vi "StandAlone_TransientDataCollection.vi"() -> ()   [LabVIEW 2019]
uses:
  <instrlib>/niScope/Controls/niScope vertical coupling.ctl
  <vilib>/Utility/file.llb/Write Delimited Spreadsheet (string).vi
  <instrlib>/niScope/Configure/Trigger/niScope Configure Trigger Software.vi
  <instrlib>/niScope/Acquire/Fetch/niScope Multi Fetch Binary 16.vi
panel:
  in  "ON/OFF":bool
  in  "Using an RF Source?":bool
  in  "power (dBm)":dbl
  in  "frequency (GHz)":dbl
  in  "Apply RF Source Changes":bool
  in  "RF Source":refnum<visa-resource-name>
  out "current limit ind":dbl
  out "Channel 0 Reference Values":dbl[](array[numeric])
  out "CHANNEL 7 NAME":string
  out "CHANNEL 6 NAME":string
  out "CHANNEL 5 NAME":string
  out "CHANNEL 4 NAME":string
  out "CHANNEL 3 NAME":string
  out "CHANNEL 2 NAME":string
  out "CHANNEL 1 NAME":string
  out "CHANNEL 0 NAME":string
  out "RUN_FOLDER":path
  out "RESTART PROGRAM SOON (DATACOLLECT)":bool
  out "Sample Rate IND":dbl
  out "Channel To Mitigate (0-7) IND":i32
  out "Collecting Data":bool
  out "RESTART PROGRAM SOON (DATASTORE)":bool
  out "Threshold Value":dbl
  out "Num Loop 4 Reset Graph":i32
  out "Channel Graph Cumulative 7":dbl[](graph)
  out "Channel Graph Cumulative 6":dbl[](graph)
  out "Channel Graph Cumulative 5":dbl[](graph)
  out "Channel Graph Cumulative 4":dbl[](graph)
  out "Channel Graph Cumulative 3":dbl[](graph)
  out "Channel Graph Cumulative 2":dbl[](graph)
  out "Channel Graph Cumulative 1":dbl[](graph)
  out "Channel Graph Cumulative 0":dbl[](graph)
  out "Channel Graph 7":dbl[](graph)
  out "Channel Graph 6":dbl[](graph)
  out "Channel Graph 5":dbl[](graph)
  out "Channel Graph 4":dbl[](graph)
  out "Channel Graph 3":dbl[](graph)
  out "Channel Graph 2":dbl[](graph)
  out "Channel Graph 1":dbl[](graph)
  out "Channel Graph 0":dbl[](graph)
  in  "Channel To Mitigate (0-7)":i32
  out "Last Point Fetched":i32
  out "Total Points Fetched":i32
  out "NUMBER SAMPLES":i32
  out "XINC":dbl
  out "Nominal Current IND":dbl
  out "Percent Threshold IND":dbl
  out "EXCEED THRESHOLD":bool
  out "EXCEED DURATION":bool
  out "Over Threshold Number":i32
  out "number of resets":i32
  out "ENABLE STATE":bool
  in  "DC Power On":bool
  in  "TRANSIENT TIME DURATION (ms)":dbl=500.0
  in  "milliseconds to wait":u32
  in  "vertical coupling":T1=1 items=["AC", "DC", "Ground"]
  in  "min record length":i32=100000
  in  "INTIALIZE SCOPE":bool
  in  "50 ohm vertical range (V)":dbl=10.0 caption="50 ohm vertical range" format="%.2f"
  in  "Channel 0 50 ohms?":bool
  out "wfm info IND":T2(array[cluster]) caption="wfm info" {"reserved2" format="%.2f"; "reserved1" format="%.2f"; "offset" format="%^.3e"; "gain" format="%^.3e"; "xIncrement" format="%^.3e"; "relativeInitialX" format="%^.3e"; "absoluteInitialX" format="%^.3e"}
  out "AUTOMITIGATION ENABLED IND":bool
  in  "AUTOMITIGATION ENABLED":bool
  out "Vertical Range (V) IND":dbl=30.0 caption="Vertical Range (V)" format="%_3g"
  out "channels IND":string="0" caption="channels"
  out "Min. Sample Rate IND":dbl=50000.0 caption="Min. Sample Rate" format="%#_6p"
  in  "Ion (ex. Kr)":string
  in  "Effective LET":string
  in  "Board Number":string
  in  "DUT":string
  in  "Beam On?":bool
  in  "Percent Threshold":dbl
  in  "Nominal Mitigation Value":dbl
  out "Number Of Channels":i32
  in  "Plot Data?":bool=TRUE
  out "CURRENTPATH":path
  out "FOLDERCREATED":bool=TRUE
  out "IndicatorOutputs":cluster{"Run Information":string, string}
  out "Latchup_or_Transient":bool
  out "BinaryRefObjects":T3
  out "OscopeParamPath":path
  out "INITIALIZED":bool
  in  "APPLYPATH":bool
  in  "INPUTPATH":path=path "C:/Campaigns/LBNL_May_2025"
  in  "Max Points per Fetch":i32=-1
  in  "channels":string="Current,Vin,Vout1,Vout2,PowerGood1_2,EN1,EN2,BeamSignal" caption="channels (comma separated)"
  in  "Oscilloscope":refnum<k15>="PXIe-5172"
  in  "Min. Sample Rate":dbl=50000.0 format="%#_6p"
  in  "Vertical Range (V)":dbl=30.0 format="%_3g"
  out "RECORDING DATA":bool
  in  "BEGIN RECORDING":bool
  out "Present Mitigation Information":string
  out "NIDCPOWER_VOLT_CONF":dbl caption="voltage level IND" format="%.6p"
  out "NIDCPOWER_CHAN_CONF":string
  in  "NIDCPOWER_VOLT":dbl caption="voltage level" format="%.6p"
  in  "NIDCPOWER_CHAN":string="0"
  in  "resource name":refnum<k15>="Slot_4_PXIe4139" caption="DC Power PSU"
  in  "CHANGE MITIGATION":bool
  in  "Mitigation":u16(ring) items=["None", "Hardware", "PowerCycle", "EnableCircuit"]
  out "FINISH PROGRAM":bool
  in  "FORCED RESET":bool
  out "POWER STATE":bool
  in  "Channels to Parallelize (if selected)":u16(ring) items=["I1+I2", "ALL", "I2+I3"]
  out "Present Channel Configuration":string
  out "Channels Configured and Values":string[][](array[string])
  in  "Combination":u16(ring) items=["OFF", "SERIES", "PARALLEL"]
  in  "PSU":refnum<visa-resource-name>="USB0::0x05E6::0x2230::802901012767010005::INSTR"
  in  "Current Limit Channel 3":dbl
  in  "Current Limit Channel 2":dbl
  in  "Current Limit Channel 1":dbl
  in  "Voltage Channel 3":dbl
  in  "Voltage Channel 2":dbl
  in  "Voltage Channel 1":dbl
  in  "stop":bool
  in  "APPLY POWER SETTINGS":bool
  in  "POWER ON":bool
  # "11 In order, name all of the channels 0-7"
  # "3 press the white arrow"
  # "10 this is the maximum. Make it smaller for better resolution"
  # "OSCILLOSCOPE BLOCK"
  # "DATA BLOCK"
  # "5 enter where the data"
  # "Use this for step three"
  # "9 if needed"
  # "12 set the scope to the configurations from steps 9-11 on device"
  # "Nothing behind here"
  # "6 enter in values before each run"
  # "need to fix this"
  # "13,16 begin recording data"
  # "1"
  # "17 end program"
  # "2"
  # "14,15 saying the beam is on or could just have the TTL logic"
  # "7 enter in values before each run"
  # "POWER BLOCK"
  # "NI DCPower"
  # "NOTE THAT VISA POWER HAS THE NI DC POWER TURN OFF AS WELL"
  # "4"
  # "Current"
  # "8 power on device"
  # "Ignore all of this"
  # "7 power on device"
  # "7 power on device"
  # "7 power on device"
  # "7 power on device"
  # "7 power on device"
  # "7 power on device"
  # "7 power on device"
  # "7 power on device"
  # "7 power on device"
  # "7 power on device"
  # "7 power on device"
  # "7 power on device"
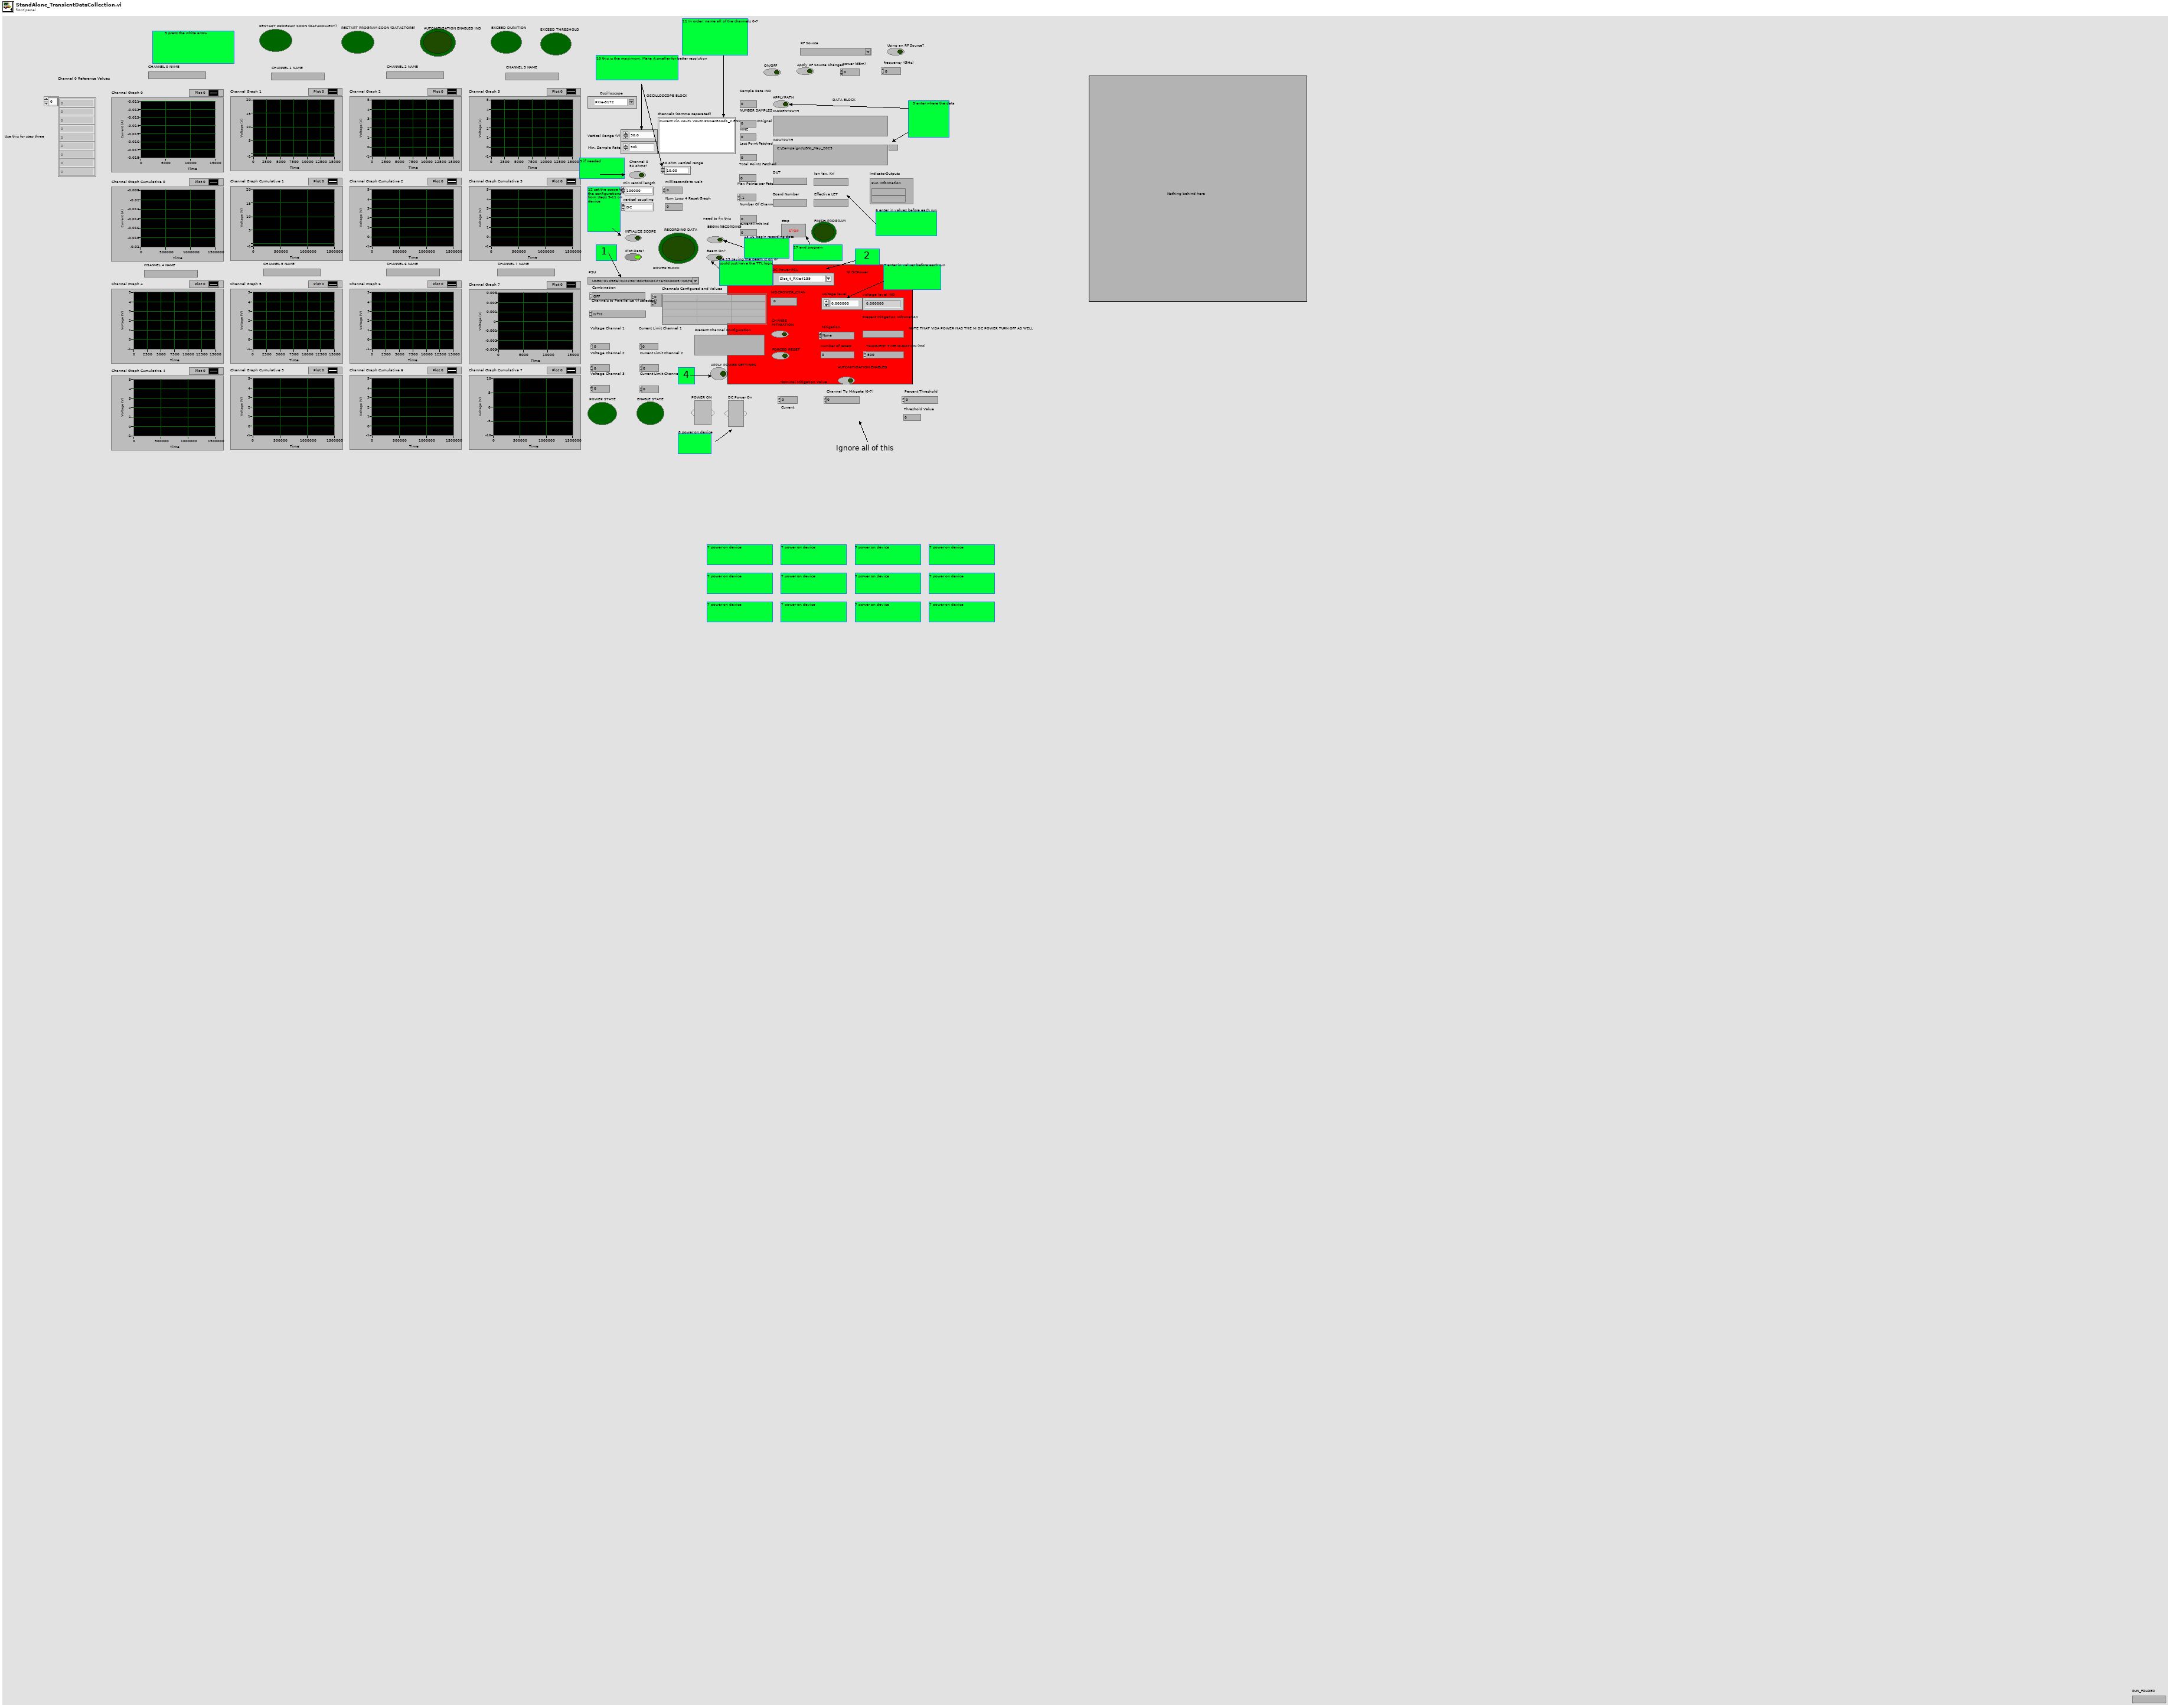
[diagram p1: front panel]
types:
  T1 = typedef "niScope vertical coupling.ctl" = i32
  T2 = cluster{"actualSamples":i32, "absoluteInitialX":dbl, "relativeInitialX":dbl, "xIncrement":dbl, "offset":dbl, "gain":dbl, "reserved1":dbl, "reserved2":dbl}[]
  T3 = cluster{"appended path":path, "refnum out":refnum<file>, "refnum out":refnum<file>, "refnum out":refnum<file>}
  T4 = cluster{"array":dbl[], "array":dbl[], "array":dbl[], "array":dbl[], "array":dbl[], "array":dbl[], "array":dbl[], "array":dbl[]}
  T5 = cluster{"wfm info":cluster{"actualSamples":i32, "absoluteInitialX":dbl, "relativeInitialX":dbl, "xIncrement":dbl, "offset":dbl, "gain":dbl, "reserved1":dbl, "reserved2":dbl}[], "wfm":i16[][], "Beam On?":bool, i32}
  T6 = enum16{"open", "replace", "create", "open or create", "replace or create", "replace or create with confirmation"}
  T7 = enum16{"big-endian, network order", "native, host order", "little-endian"}
  T8 = cluster{"wfm info":cluster{"actualSamples":i32, "absoluteInitialX":dbl, "relativeInitialX":dbl, "xIncrement":dbl, "offset":dbl, "gain":dbl, "reserved1":dbl, "reserved2":dbl}[], "wfm":i16[][]}
  T9 = cluster{"actualSamples":i32, "absoluteInitialX":dbl, "relativeInitialX":dbl, "xIncrement":dbl, "offset":dbl, "gain":dbl, "reserved1":dbl, "reserved2":dbl}
  T10 = cluster{"AUTOMITIGATION ENABLED IND":bool, "Present Mitigation Information":string}
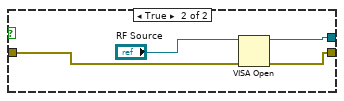
[diagram p2: hidden frame]
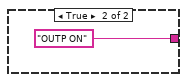
[diagram p4: hidden frame]
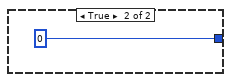
[diagram p5: hidden frame]
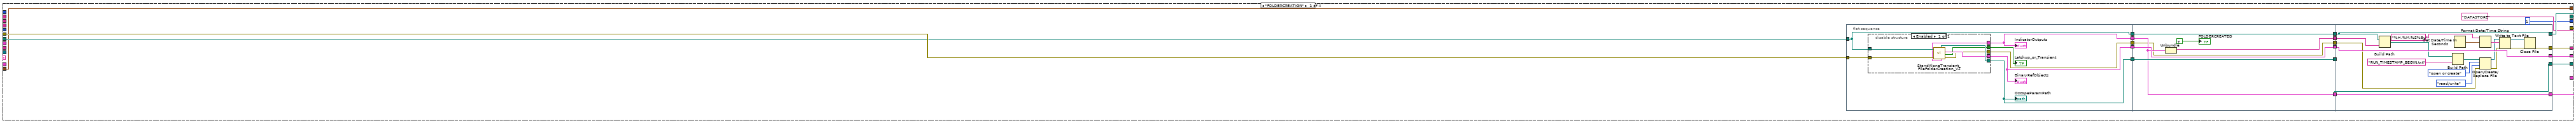
[diagram p6: hidden frame]
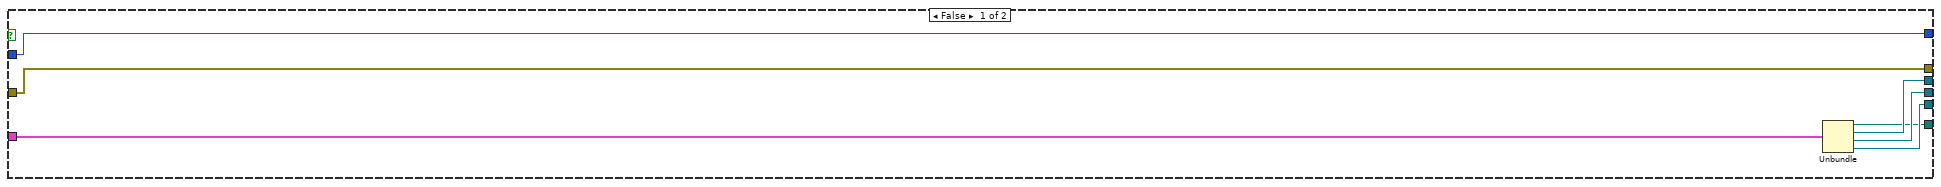
[diagram p7: hidden frame]
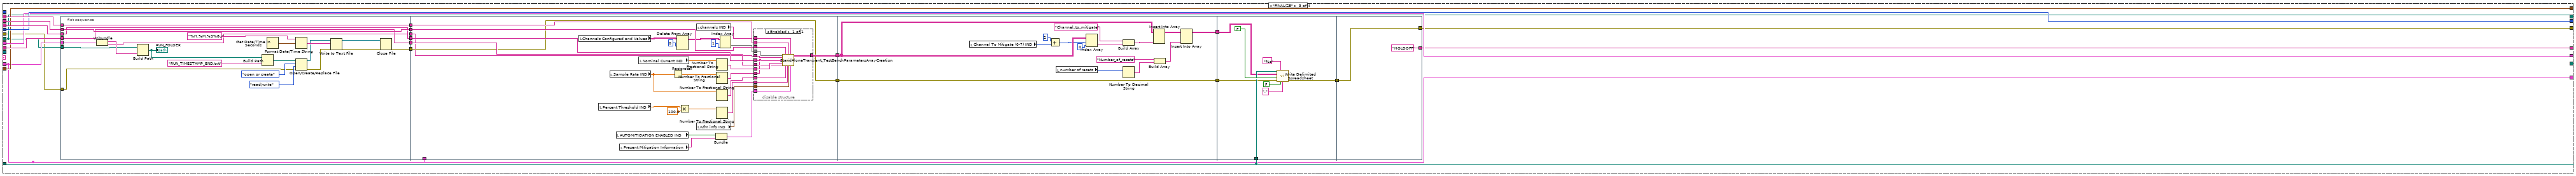
[diagram p10: hidden frame]
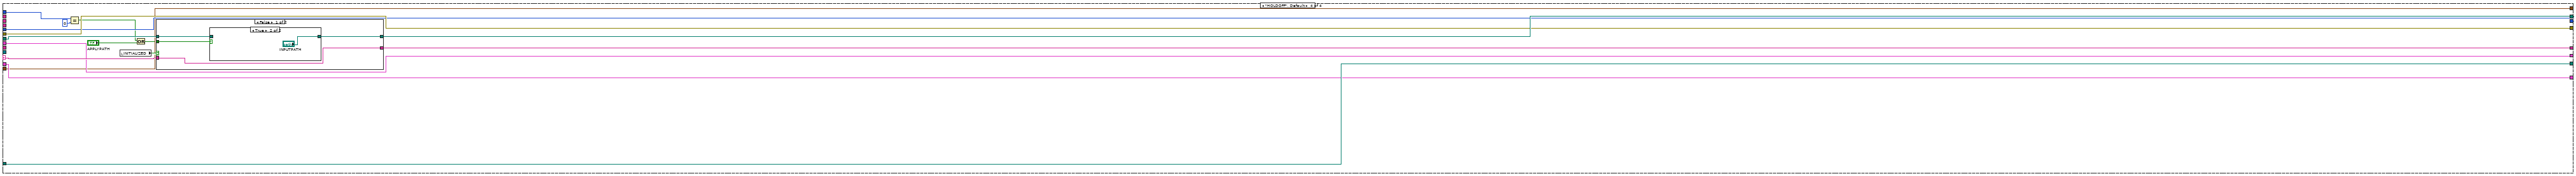
[diagram p11: hidden frame]
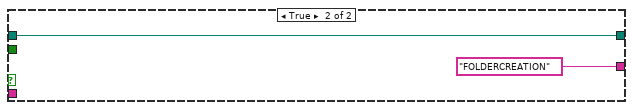
[diagram p13: hidden frame]
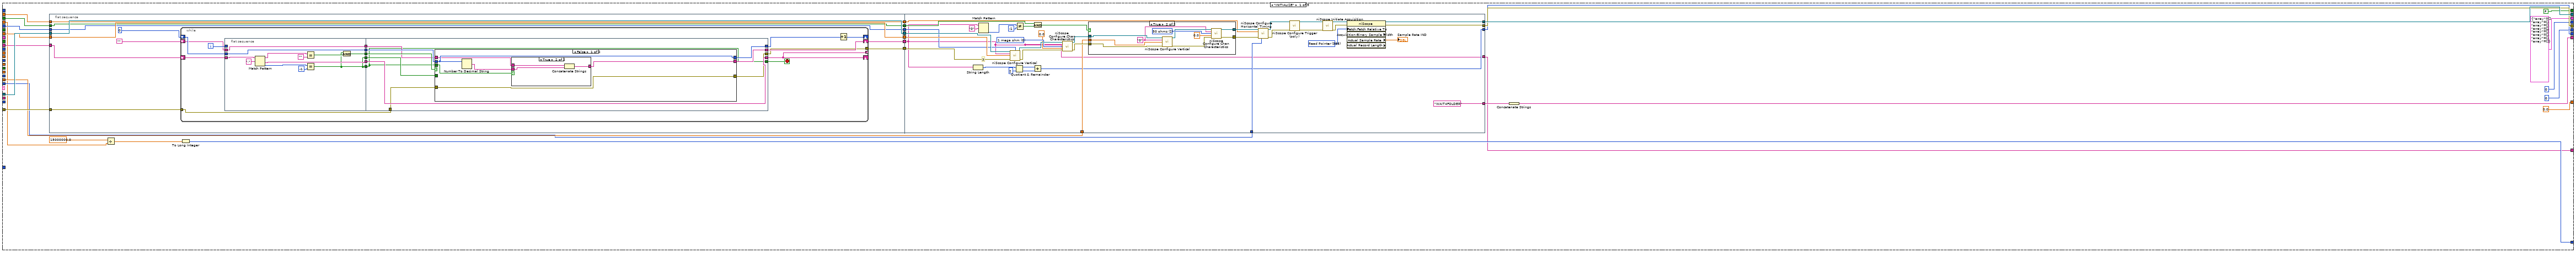
[diagram p14: hidden frame]
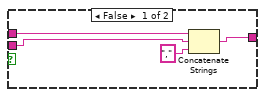
[diagram p15: hidden frame]
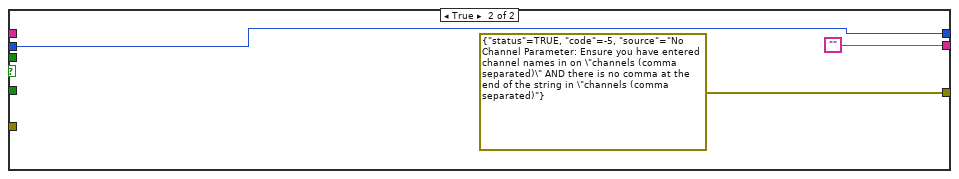
[diagram p16: hidden frame]
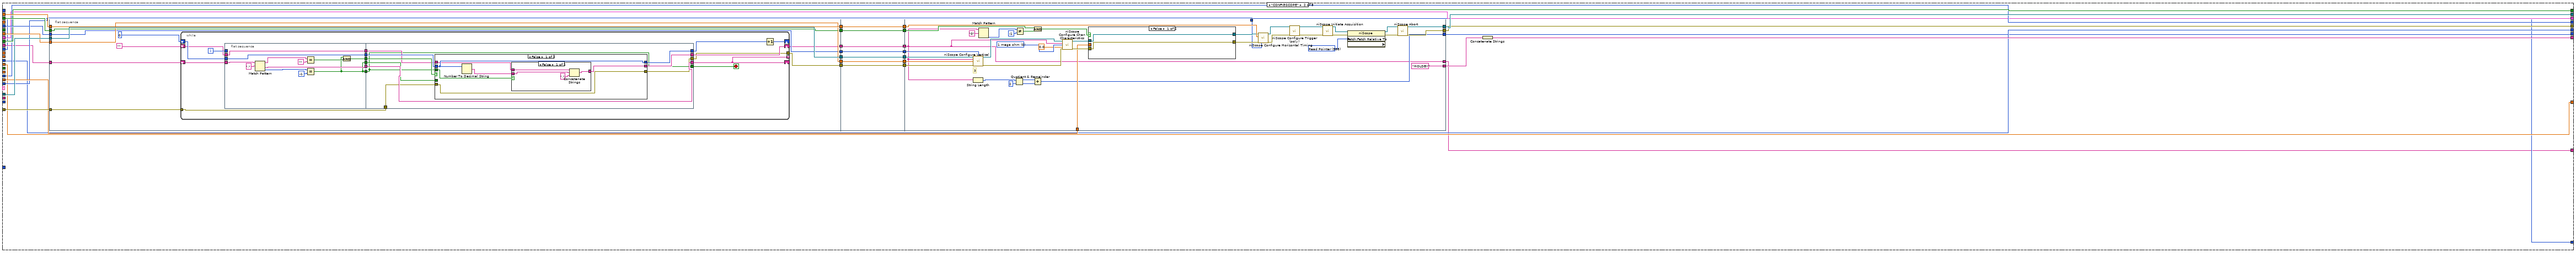
[diagram p18: hidden frame]
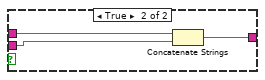
[diagram p19: hidden frame]
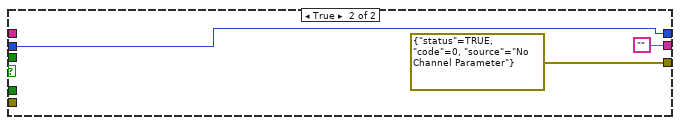
[diagram p20: hidden frame]
diagram:
  # "C:\\NULL"
  # "Moved Graph outputting into the collection to make it closer to live. Moved queueing to after the software reading as well so we can put everything inside the queueing element for better synchronization"
  # "Moved Software reading to the collection terminal to make the processing faster"
  n1 = flat-sequence {
    tunnel: [w10] -> w3
    tunnel: [w9] -> w2
    tunnel: w3 -> [w49]
    tunnel: w2 -> [w50]
    tunnel: [w16] -> w1
    frame #0 {
      w11 = FALSE  # Reset Device
      n2 = local write "number of resets"(0 ("number of resets")) -> ()
      n3 = local write "NIDCPOWER_VOLT_CONF"(0.0 ("NIDCPOWER_VOLT_CONF")) -> ()
      n4 = local write "Channel To Mitigate (0-7) IND"(0) -> ()
      n5 = local write "FINISH PROGRAM"(FALSE) -> ()
      n6 = local write "Collecting Data"(FALSE ("Collecting Data")) -> ()
      n7 = local write "EXCEED DURATION"(FALSE) -> ()
      n8 = local write "FOLDERCREATED"(FALSE) -> ()
      n9 = local write "NIDCPOWER_CHAN_CONF"("0" ("NIDCPOWER_CHAN_CONF")) -> ()
      n10 = call <instrlib>:"niScope Initialize.vi"("resource name"="Oscilloscope", "reset device"=w11) -> ("instrument handle"=w9:refnum<k15>, "error out"=w10:errorcluster)  [unwired: 12 in]
    }
    frame #1 {
      (unwired) T8 {"wfm info"=[], "wfm"=[]} ("cluster")
      # "OVERTHRESHOLD"
      # "INSIDE TRANSIENT"
      # "INITIAL TIME STAMP INSIDE TRANSIENT"
      # "TOTAL POINTS COLLECTED"
      # "INITIAL\nTIME\nSTAMP \nINSIDE \nTRANSIENT"
      # "INSIDE TRANSIENT"
      # "Overthreshold counter"
      # "Capture Number"
      # "MAY WANT TO MAKE THE CONDITIONAL COMPONENT A SUBVI IN ITSELF"
      n11 = Obtain Queue(element data type=T5 {"wfm info"=[], "wfm"=[], "Beam On?"=FALSE, 0} ("cluster"), error in (no error)=w49) -> (queue out=w29:refnum<queue>, error out=w25:errorcluster)  [unwired: 3 in, 1 out]
      n12 = case shown="False" "Using an RF Source?" {
        tunnel: w25 -> [w60 w65]
        tunnel: [w60 w64] -> w24
        tunnel: [refnum<visa-resource-name> refnum ("RF Source") w62] -> w23
        frame False {
        }
        frame True {
          n13 = VISA Open(error in (no error)=w65, VISA resource name="RF Source") -> (VISA resource name=w62:refnum<visa-resource-name>, error out=w64:errorcluster)  [unwired: 3 in]
        }
      }
      n14 = while {
        shift-right: [w93] -> _
        shift-left: path "C:/NULL" ("base path") -> [w92]
        shift-right: [w91] -> _
        shift-left: "HOLDOFF" -> [w94]
        shift-right: [w90] -> w19
        shift-left: w24 -> [w70]
        shift-right: [w89] -> _
        shift-left: path "" ("OscopeParamPath") -> [w86]
        shift-right: [w88] -> _
        shift-left: T3 {"appended path"=path "", "refnum out"=refnum, "refnum out"=refnum, "refnum out"=refnum} ("BinaryRefObjects") -> [w85]
        shift-right: [w87] -> _
        shift-left: cluster{"name or relative path":string, string} {"name or relative path"="", ""} ("IndicatorOutputs") -> [w84]
        tunnel: w29 -> [w81]
        shift-right: [w82] -> _
        shift-left: 0 -> [w83]
        shift-right: [w75] -> _
        shift-left: T2 [] ("wfm info") -> [w76]
        tunnel: w23 -> [w68]
        tunnel: [w66] -> w17
        i -> [w72]
        stop <- w95 stop-if-true
        n15 = case shown="True" "Apply RF Source Changes" {
          tunnel: w70 -> [w97 w109]
          tunnel: [w97 w102] -> w69
          tunnel: w68 -> [w96 w108]
          tunnel: [w96 w100] -> w66
          frame False {
          }
          frame True {
            n16 = Multiply(x=1000000000.0 ("y"), y="frequency (GHz)") -> (x*y=w106:dbl)
            n17 = Number To Fractional String(number=w106) -> (F-format string=w117:string)  [unwired: 3 in]
            n18 = case shown="False" "ON/OFF" {
              tunnel: ["OUTP OFF" ("write buffer") "OUTP ON" ("write buffer")] -> w104
              frame False {
              }
              frame True {
              }
            }
            n19 = Number To Fractional String(number="power (dBm)") -> (F-format string=w112:string)  [unwired: 3 in]
            n20 = Concatenate Strings("freq " ("string"), w117) -> (w116:string)
            n21 = Concatenate Strings("pow " ("string"), w112) -> (w114:string)
            n22 = VISA Write(VISA resource name=w108, write buffer=w116, error in (no error)=w109) -> (VISA resource name out=w113:refnum<visa-resource-name>, error out=w110:errorcluster)  [unwired: 1 out]
            n23 = VISA Write(VISA resource name=w113, write buffer=w114, error in (no error)=w110) -> (VISA resource name out=w101:refnum<visa-resource-name>, error out=w103:errorcluster)  [unwired: 1 out]
            n24 = VISA Write(VISA resource name=w101, write buffer=w104, error in (no error)=w103) -> (VISA resource name out=w100:refnum<visa-resource-name>, error out=w102:errorcluster)  [unwired: 1 out]
          }
        }
        n25 = Greater?(x=w72, y=2100000000) -> (0:w73:bool)
        n26 = case shown="False" w73 {
          tunnel: [w120 0] -> w71
          tunnel: w72 -> [w120 _]
          frame False {
          }
          frame True {
          }
        }
        n27 = case shown="\"DATASTORE\"" w94 {
          selector: w94 -> [_ w221 _ w599]
          tunnel: [w139 w232 w479 w602] -> w93
          tunnel: w92 -> [w141 w232 w479 w603]
          tunnel: ["DATASTORE" w220 w493 w600] -> w91
          tunnel: w69 -> [w142 w227 w478 w598]
          tunnel: [w122 w200 w489 w598] -> w90
          tunnel: [w137 w192 w491 w597] -> w89
          tunnel: [w135 w194 w494 w596] -> w88
          tunnel: [w133 w193 w480 w595] -> w87
          tunnel: w86 -> [_ w192 w491 w597]
          tunnel: w85 -> [_ w224 w494 w596]
          tunnel: w84 -> [_ w193 w480 w595]
          tunnel: w71 -> [_ w231 _ w589]
          tunnel: w83 -> [_ w230 w495 w594]
          tunnel: [1 w204 w495 w594] -> w82
          tunnel: w81 -> [_ w223 _ _]
          tunnel: "DUT" -> [_ _ w496 _]
          tunnel: "Board Number" -> [_ _ w497 _]
          tunnel: "Effective LET" -> [_ _ w499 _]
          tunnel: "Ion (ex. Kr)" -> [_ _ w498 _]
          tunnel: [w130 w190 w492 w593] -> w75
          tunnel: w76 -> [w130 w189 w492 w593]
          frame "FOLDERCREATION" {
            n28 = flat-sequence {
              tunnel: w142 -> [w143]
              tunnel: w141 -> [w149]
              tunnel: [w149] -> w140
              tunnel: [w148] -> w136
              tunnel: [w147] -> w134
              tunnel: [w145] -> w132
              tunnel: [w144] -> w123
              tunnel: w140 -> [w162]
              tunnel: w136 -> [w161]
              tunnel: w134 -> [w160]
              tunnel: w132 -> [w159]
              tunnel: [w162] -> w129
              tunnel: [w161] -> w128
              tunnel: [w160] -> w127
              tunnel: [w159] -> w126
              tunnel: [w158] -> w125
              tunnel: [w157] -> w124
              tunnel: w123 -> [w157]
              tunnel: [w180] -> w133
              tunnel: [w181] -> w135
              tunnel: [w182] -> w137
              tunnel: [w167] -> w139
              tunnel: w129 -> [w167]
              tunnel: w128 -> [w182]
              tunnel: w127 -> [w181]
              tunnel: w126 -> [w180]
              tunnel: w125 -> [w166]
              tunnel: [w165] -> w122
              tunnel: w124 -> [w164]
              frame #0 {
                n29 = disable-structure shown="Enabled" {
                  disable-tunnel: w149 -> [w155]
                  disable-tunnel: [w154] -> w148
                  disable-tunnel: [w153] -> w147
                  disable-tunnel: [w152] -> w146
                  disable-tunnel: [w150] -> w145
                  disable-tunnel: [w151] -> w144
                  disable-tunnel: w143 -> [w156]
                  frame Enabled {
                    n30 = call "StandAloneTransient_FileFolderCreation_V2.vi"("error in (no error)"=w156, "base path"=w155) -> ("error out"=w151:errorcluster, "Latchup_or_Transient"=w152:bool, "BinaryRefObjects"=w153:T3, "IndicatorOutputs"=w150:cluster{"name or relative path":string, string}, "OscopeParamPath"=w154:path)  [unwired: 4 in, 1 out]
                  }
                }
                "OscopeParamPath" <- w148
                "BinaryRefObjects" <- w147
                "Latchup_or_Transient" <- w146
                "IndicatorOutputs" <- w145
              }
              frame #1 {
                n31 = Unbundle(w159) -> ("name or relative path"=w158:string)  [unwired: 1 out]
                "FOLDERCREATED" <- TRUE
              }
              frame #2 {
                n32 = Build Path(base path=w167, name or relative path=w166) -> (appended path=w179:path)
                n33 = Build Path(base path=w179, name or relative path="RUN_TIMESTAMP_BEGIN.txt") -> (appended path=w174:path)
                n34 = Get Date/Time In Seconds() -> (seconds since 1Jan1904=w177:timestamp)
                n35 = Format Date/Time String(time format string (%c)="%H.%M.%S%8u", seconds (now)=w177) -> (date/time string=w178:string)  [unwired: 1 in]
                n36 = Open/Create/Replace File(file path (use dialog)=w174, error in=w164, operation (0:open)=T6."open or create", access (0:read/write)=enum16{"read/write", "read-only", "write-only"}."read/write") -> (refnum out=w172:refnum<file>, error out=w173:errorcluster)  [unwired: 2 in, 1 out]
                n37 = Write to Text File(file (use dialog)=w172, text=w178, error in=w173) -> (refnum out=w176:refnum<file>, error out=w175:errorcluster)  [unwired: 1 in, 1 out]
                n38 = Close File(refnum=w176, error in=w175) -> (error out=w165:errorcluster)  [unwired: 1 out]
              }
            }
          }
          frame "DATASTORE" {
            # "IMPEMENT THE ACTUAL DATASTORE USING THE ENQUEING THAT WE KNOW FROM OLD DATACOLLECTION VIS"
            n39 = flat-sequence {
              tunnel: w231 -> [w233]
              tunnel: w230 -> [w235]
              tunnel: [w237] -> w229
              tunnel: [w236] -> w228
              tunnel: w227 -> [w236]
              tunnel: [w235] -> w226
              tunnel: [w234] -> w225
              tunnel: w224 -> [w234]
              tunnel: w229 -> [w252]
              tunnel: w228 -> [w251]
              tunnel: w226 -> [w249]
              tunnel: w225 -> [w248]
              tunnel: [w250] -> w188
              tunnel: [w247] -> w187
              tunnel: [w246] -> w186
              tunnel: [w245] -> w185
              tunnel: [w244] -> w184
              tunnel: [w243] -> w183
              tunnel: w223 -> [w338]
              tunnel: [w333] -> w222
              tunnel: [w331] -> w218
              tunnel: [w329] -> w216
              tunnel: [w328] -> w213
              tunnel: [w327] -> w211
              tunnel: [w326] -> w209
              tunnel: [w325] -> w207
              tunnel: [w324] -> w205
              tunnel: [w323] -> w202
              tunnel: w183 -> [w323]
              tunnel: w184 -> [w324]
              tunnel: w185 -> [w328]
              tunnel: w186 -> [w327]
              tunnel: w187 -> [w326]
              tunnel: w188 -> [w337]
              tunnel: w222 -> [w352]
              tunnel: w221 -> [w351]
              tunnel: [w350] -> w220
              tunnel: [w349] -> w219
              tunnel: w218 -> [w349]
              tunnel: [TRUE] -> w217
              tunnel: w216 -> [_]
              tunnel: [w348] -> w215
              tunnel: [w347] -> w214
              tunnel: w213 -> [w347]
              tunnel: [w346] -> w212
              tunnel: w211 -> [w346]
              tunnel: [w345] -> w210
              tunnel: w209 -> [w345]
              tunnel: [w344] -> w208
              tunnel: w207 -> [w344]
              tunnel: [w343] -> w206
              tunnel: w205 -> [w343]
              tunnel: [w342] -> w203
              tunnel: w202 -> [w342]
              tunnel: w219 -> [w369]
              tunnel: w217 -> [w368]
              tunnel: w215 -> [w367]
              tunnel: w214 -> [w366]
              tunnel: w212 -> [w364]
              tunnel: w210 -> [w363]
              tunnel: w208 -> [w365]
              tunnel: w206 -> [w362]
              tunnel: w203 -> [w357]
              tunnel: [w362] -> w201
              tunnel: [w361] -> w199
              tunnel: [w360] -> w198
              tunnel: [w359] -> w197
              tunnel: [w358] -> w196
              tunnel: [w357] -> w195
              tunnel: w189 -> [w356]
              tunnel: [w355] -> w191
              tunnel: [w475] -> w204
              tunnel: w201 -> [w475]
              tunnel: [w474] -> w200
              tunnel: w199 -> [w474]
              tunnel: w198 -> [w473]
              tunnel: w197 -> [w472]
              tunnel: w196 -> [w471]
              tunnel: w195 -> [w470]
              tunnel: [w469] -> w194
              tunnel: w191 -> [w468]
              tunnel: [w468] -> w190
              frame #0 {
                # "Iterations of the buffer loop until the next file is made. Tradeoff: Larger = worry about overflow \nSmaller = smaller files to process and less likelihood of overflowing, but more to push through the reading code which is bottlenecked by the write to csv code"
                n40 = Quotient & Remainder(x=w233, y=100) -> (x-y*floor(x/y)=w240:i32, floor(x/y)=w241:i32)
                n41 = Equal To 0?(x=w240) -> (x = 0?=w238:bool)
                n42 = Not Equal To 0?(x=w241) -> (x != 0?=w239:bool)
                n43 = And(x=w238, y=w239) -> (x .and. y?=w237:bool)
              }
              frame #1 {
                n44 = case shown="True" w252 {
                  tunnel: w251 -> [w259 w276]
                  tunnel: [w259 w263] -> w250
                  tunnel: w249 -> [w254 w275]
                  tunnel: w248 -> [w258 w274]
                  tunnel: [w255 w266] -> w247
                  tunnel: [w256 w265] -> w246
                  tunnel: [w257 w264] -> w245
                  tunnel: [w254 w262] -> w244
                  tunnel: [w253 w261] -> w243
                  frame False {
                    n45 = Unbundle(w258) -> ("appended path"=w253:path, "refnum out"=w257:refnum<file>, "refnum out"=w256:refnum<file>, "refnum out"=w255:refnum<file>)
                  }
                  frame True {
                    n46 = flat-sequence {
                      tunnel: w276 -> [w283]
                      tunnel: w275 -> [w299]
                      tunnel: w274 -> [w298]
                      tunnel: [w285] -> w273
                      tunnel: [w284] -> w272
                      tunnel: [w283] -> w271
                      tunnel: [w282] -> w270
                      tunnel: [w281] -> w269
                      tunnel: [w280] -> w268
                      tunnel: [w279] -> w267
                      tunnel: [w278] -> w262
                      tunnel: [w277] -> w260
                      tunnel: w273 -> [w320]
                      tunnel: w272 -> [w319]
                      tunnel: w271 -> [w314]
                      tunnel: w270 -> [w308]
                      tunnel: w269 -> [w307]
                      tunnel: w268 -> [w306]
                      tunnel: w267 -> [w305]
                      tunnel: [w304] -> w266
                      tunnel: [w303] -> w265
                      tunnel: [w302] -> w264
                      tunnel: [w301] -> w263
                      tunnel: [w300] -> w261
                      tunnel: w260 -> [w300]
                      frame #0 {
                        n47 = Increment(x=w299) -> (x+1=w278:i32)
                        n48 = Number To Decimal String(number=w278) -> (decimal integer string=w288:string)  [unwired: 1 in]
                        n49 = Number To Decimal String(number=w278) -> (decimal integer string=w291:string)  [unwired: 1 in]
                        n50 = Number To Decimal String(number=w278) -> (decimal integer string=w295:string)  [unwired: 1 in]
                        n51 = Concatenate Strings("SamplePerCap_", w288, ".sbdf" ("string")) -> (w286:string)
                        n52 = Concatenate Strings("WaveformData_", w291, ".sbdf" ("string")) -> (w290:string)
                        n53 = Concatenate Strings("SampleData_", w295, ".sbdf" ("string")) -> (w294:string)
                        n54 = Unbundle(w298) -> ("appended path"=w277:path, "refnum out"=w284:refnum<file>, "refnum out"=w280:refnum<file>, "refnum out"=w279:refnum<file>)
                        n55 = Build Path(base path=w277, name or relative path=w286) -> (appended path=w281:path)
                        n56 = Build Path(base path=w277, name or relative path=w290) -> (appended path=w282:path)
                        n57 = Build Path(base path=w277, name or relative path=w294) -> (appended path=w285:path)
                      }
                      frame #1 {
                        n58 = Close File(refnum=w319, error in=w314) -> (error out=w313:errorcluster)  [unwired: 1 out]
                        n59 = Open/Create/Replace File(file path (use dialog)=w320, error in=w313, operation (0:open)=T6."open or create", access (0:read/write)=enum16{"read/write", "read-only", "write-only"}."read/write") -> (refnum out=w302:refnum<file>, error out=w312:errorcluster)  [unwired: 2 in, 1 out]
                        n60 = Close File(refnum=w306, error in=w312) -> (error out=w311:errorcluster)  [unwired: 1 out]
                        n61 = Open/Create/Replace File(file path (use dialog)=w308, error in=w311, operation (0:open)=T6."open or create", access (0:read/write)=enum16{"read/write", "read-only", "write-only"}."read/write") -> (refnum out=w303:refnum<file>, error out=w310:errorcluster)  [unwired: 2 in, 1 out]
                        n62 = Close File(refnum=w305, error in=w310) -> (error out=w309:errorcluster)  [unwired: 1 out]
                        n63 = Open/Create/Replace File(file path (use dialog)=w307, error in=w309, operation (0:open)=T6."open or create", access (0:read/write)=enum16{"read/write", "read-only", "write-only"}."read/write") -> (refnum out=w304:refnum<file>, error out=w301:errorcluster)  [unwired: 2 in, 1 out]
                      }
                    }
                  }
                }
              }
              frame #2 {
                n64 = local read "RECORDING DATA"() -> (w336:bool)
                n65 = Get Queue Status(queue=w338, error in (no error)=w337) -> (queue out=w339:refnum<queue>, error out=w332:errorcluster, # elements in queue=w330:i32)  [unwired: 1 in, 5 out]
                n66 = Equal To 0?(x=w330) -> (x = 0?=w334:bool)
                n67 = Greater Than 0?(x=w330) -> (x > 0?=w329:bool)
                n68 = Not(x=w336) -> (.not. x?=w335:bool)
                n69 = And(x=w334, y=w335) -> (x .and. y?=w333:bool)
                n70 = Dequeue Element(queue=w339, timeout in ms (-1)=100, error in (no error)=w332) -> (element=w331:T5, error out=w325:errorcluster)  [unwired: 2 out]
              }
              frame #3 {
                n71 = case shown="True" w352 {
                  tunnel: [w353 "FINALIZE"] -> w350
                  tunnel: w351 -> [w353 _]
                  frame False {
                  }
                  frame True {
                  }
                }
                n72 = local read "Number Of Channels"() -> (w348:i32)
              }
              frame #4 {
                n73 = case shown="True" w368 {
                  tunnel: w369 -> [_ w406]
                  tunnel: w367 -> [_ w404]
                  tunnel: w366 -> [w372 w402]
                  tunnel: w365 -> [w371 w401]
                  tunnel: w364 -> [w373 w395]
                  tunnel: w363 -> [w374 w394]
                  tunnel: [w371 w389] -> w361
                  tunnel: [w374 w388] -> w360
                  tunnel: [w373 w387] -> w359
                  tunnel: [w372 w385] -> w358
                  tunnel: w356 -> [w370 _]
                  tunnel: [w370 w382] -> w355
                  frame False {
                  }
                  frame True {
                    n74 = Unbundle(w406) -> ("wfm info"=w382:T2, "wfm"=w405:i16[][], "Beam On?"=w380:bool, w379:i32)
                    n75 = flat-sequence {
                      tunnel: [w413] -> w403
                      tunnel: [w414] -> w399
                      tunnel: [w411] -> w381
                      tunnel: [w409] -> w378
                      tunnel: [w408] -> w377
                      tunnel: w379 -> [w409]
                      tunnel: w380 -> [w408]
                      tunnel: w401 -> [w407]
                      tunnel: w405 -> [w414]
                      tunnel: w382 -> [w412]
                      tunnel: w404 -> [_]
                      tunnel: [w407] -> w376
                      tunnel: w403 -> [w420]
                      tunnel: [w427] -> w400
                      tunnel: w399 -> [w427]
                      tunnel: [w426] -> w397
                      tunnel: [w425] -> w391
                      tunnel: w381 -> [w421]
                      tunnel: w378 -> [w417]
                      tunnel: w377 -> [w416]
                      tunnel: w376 -> [w415]
                      tunnel: [w415] -> w375
                      tunnel: w402 -> [w438]
                      tunnel: w400 -> [w437]
                      tunnel: [w436] -> w398
                      tunnel: w397 -> [w436]
                      tunnel: [w435] -> w396
                      tunnel: [w434] -> w392
                      tunnel: w391 -> [w434]
                      tunnel: [w433] -> w383
                      tunnel: w375 -> [w432]
                      tunnel: w398 -> [w450]
                      tunnel: w396 -> [w449]
                      tunnel: w395 -> [w448]
                      tunnel: [w447] -> w393
                      tunnel: w392 -> [w447]
                      tunnel: [w446] -> w390
                      tunnel: [w445] -> w386
                      tunnel: [w444] -> w384
                      tunnel: w383 -> [w444]
                      tunnel: w394 -> [w462]
                      tunnel: w393 -> [w461]
                      tunnel: w390 -> [w460]
                      tunnel: [w459] -> w389
                      tunnel: [w458] -> w388
                      tunnel: [w457] -> w387
                      tunnel: w386 -> [w457]
                      tunnel: [w456] -> w385
                      tunnel: w384 -> [w456]
                      frame #0 {
                        n76 = local read "number of resets"() -> (w413:i32)
                        n77 = Index Array(array=w412, index=0) -> (element=w411:T9)
                      }
                      frame #1 {
                        # "0. AbsoluteInitialX\n1. Xincrement\n2. Beam On? (1 yes, 0 no)\n3. Index of Maximum\n4. Rolling Transient Counter"
                        n78 = Boolean To (0,1)(Boolean=w416) -> (0, 1=w431:i16)
                        n79 = Unbundle(w421) -> ("actualSamples"=w425:i32, "absoluteInitialX"=w419:dbl, "xIncrement"=w418:dbl)  [unwired: 5 out]
                        n80 = To Double Precision Float(number=w417) -> (double precision float=w428:dbl)
                        n81 = To Double Precision Float(number=w420) -> (double precision float=w429:dbl)
                        n82 = Round To Nearest(number=w428) -> (nearest integer value=w422:dbl)
                        n83 = Round To Nearest(number=w429) -> (nearest integer value=w423:dbl)
                        n84 = To Double Precision Float(number=w431) -> (double precision float=w430:dbl)
                        n85 = Round To Nearest(number=w430) -> (nearest integer value=w424:dbl)
                        n86 = Build Array(w419, w418, w424, w422, w423) -> (w426:dbl[])
                      }
                      frame #2 {
                        n87 = Set File Position(refnum=w438, from (0:start)=enum16{"start", "end", "current"}."current", error in=w432) -> (refnum out=w442:refnum<file>, error out=w443:errorcluster)  [unwired: 1 in]
                        n88 = Write to Binary File(file (use dialog)=w442, data=w437, error in=w443, 5:FALSE ("prepend array or string size? (T)"), 9:T7."little-endian" ("byte order (0:big-endian, network order)")) -> (refnum out=w433:refnum<file>, error out=w435:errorcluster)  [unwired: 1 in, 1 out]
                      }
                      frame #3 {
                        n89 = Set File Position(refnum=w448, from (0:start)=enum16{"start", "end", "current"}."current", error in=w449) -> (refnum out=w454:refnum<file>, error out=w455:errorcluster)  [unwired: 1 in]
                        n90 = Write to Binary File(file (use dialog)=w454, data=w450, error in=w455, 5:FALSE ("prepend array or string size? (T)"), 9:T7."little-endian" ("byte order (0:big-endian, network order)")) -> (refnum out=w445:refnum<file>, error out=w446:errorcluster)  [unwired: 1 in, 1 out]
                      }
                      frame #4 {
                        n91 = Set File Position(refnum=w462, from (0:start)=enum16{"start", "end", "current"}."current", error in=w460) -> (refnum out=w466:refnum<file>, error out=w467:errorcluster)  [unwired: 1 in]
                        n92 = Write to Binary File(file (use dialog)=w466, data=w461, error in=w467, 5:FALSE ("prepend array or string size? (T)"), 9:T7."little-endian" ("byte order (0:big-endian, network order)")) -> (refnum out=w458:refnum<file>, error out=w459:errorcluster)  [unwired: 1 in, 1 out]
                      }
                    }
                  }
                }
              }
              frame #5 {
                n93 = Bundle("appended path"=w470, "refnum out"=w471, "refnum out"=w472, "refnum out"=w473) -> (w469:T3)  [unwired: 1 in]
              }
            }
          }
          frame "FINALIZE" {
            n94 = flat-sequence {
              tunnel: w496 -> [w518]
              tunnel: w497 -> [w519]
              tunnel: w498 -> [w520]
              tunnel: w499 -> [w521]
              tunnel: [w521] -> w484
              tunnel: [w520] -> w483
              tunnel: [w519] -> w482
              tunnel: [w518] -> w481
              tunnel: w480 -> [w506]
              tunnel: w479 -> [w504]
              tunnel: w478 -> [w502]
              tunnel: [w501] -> w477
              tunnel: [w500] -> w476
              tunnel: w480 -> [_]
              tunnel: [w523] -> w488
              tunnel: [w531] -> w486
              tunnel: w484 -> [w548]
              tunnel: w483 -> [w547]
              tunnel: w482 -> [w546]
              tunnel: w481 -> [w545]
              tunnel: w477 -> [w523]
              tunnel: w476 -> [w522]
              tunnel: w488 -> [w577]
              tunnel: [w577] -> w487
              tunnel: w486 -> [w573]
              tunnel: [w563] -> w485
              tunnel: w491 -> [w582]
              tunnel: w487 -> [w580]
              tunnel: [w579] -> w490
              tunnel: w485 -> [w578]
              tunnel: ["HOLDOFF"] -> w493
              tunnel: w490 -> [w586]
              tunnel: [w586] -> w489
              frame #0 {
                n95 = Unbundle(w506) -> ("name or relative path"=w505:string, w500:string)
                n96 = Build Path(base path=w504, name or relative path=w505) -> (appended path=w503:path)
                "RUN_FOLDER" <- w503
                n97 = Build Path(base path=w503, name or relative path="RUN_TIMESTAMP_END.txt") -> (appended path=w512:path)
                n98 = Get Date/Time In Seconds() -> (seconds since 1Jan1904=w516:timestamp)
                n99 = Format Date/Time String(time format string (%c)="%H.%M.%S%8u", seconds (now)=w516) -> (date/time string=w517:string)  [unwired: 1 in]
                n100 = Open/Create/Replace File(file path (use dialog)=w512, error in=w502, operation (0:open)=T6."open or create", access (0:read/write)=enum16{"read/write", "read-only", "write-only"}."read/write") -> (refnum out=w511:refnum<file>, error out=w514:errorcluster)  [unwired: 2 in, 1 out]
                n101 = Write to Text File(file (use dialog)=w511, text=w517, error in=w514) -> (refnum out=w513:refnum<file>, error out=w515:errorcluster)  [unwired: 1 in, 1 out]
                n102 = Close File(refnum=w513, error in=w515) -> (error out=w501:errorcluster)  [unwired: 1 out]
              }
              frame #1 {
                n103 = local read "Channels Configured and Values"() -> (w536:string[][])
                n104 = local read "Percent Threshold IND"() -> (w525:dbl)
                n105 = local read "Sample Rate IND"() -> (w530:dbl)
                n106 = local read "AUTOMITIGATION ENABLED IND"() -> (w542:bool)
                n107 = local read "Present Mitigation Information"() -> (w541:string)
                n108 = local read "Nominal Current IND"() -> (w527:dbl)
                n109 = Reciprocal(x=w530) -> (1/x=w539:dbl)
                n110 = Delete From Array(array=w536, index (row)=0) -> (array with subset deleted=w534:string[][])  [unwired: 2 in, 1 out]
                n111 = Multiply(x=w525, y=100.0) -> (x*y=w524:dbl)
                n112 = local read "channels IND"() -> (w529:string)
                n113 = local read "wfm info IND"() -> (w528:T2)
                n114 = Bundle("AUTOMITIGATION ENABLED IND"=w542, "Present Mitigation Information"=w541) -> (w540:T10)  [unwired: 1 in]
                n115 = Number To Fractional String(number=w527) -> (F-format string=w537:string)  [unwired: 3 in]
                n116 = Number To Fractional String(number=w539) -> (F-format string=w538:string)  [unwired: 3 in]
                n117 = Number To Fractional String(number=w530) -> (F-format string=w543:string)  [unwired: 3 in]
                n118 = Number To Fractional String(number=w524) -> (F-format string=w544:string)  [unwired: 3 in]
                n119 = Index Array(array=w534, index (col)=1 ("disabled index (col)")) -> (element=w532:string[])  [unwired: 1 in]
                n120 = disable-structure shown="Enabled" {
                  disable-tunnel: w548 -> [w561]
                  disable-tunnel: w547 -> [w560]
                  disable-tunnel: w546 -> [w556]
                  disable-tunnel: w545 -> [w555]
                  disable-tunnel: w544 -> [w551]
                  disable-tunnel: w543 -> [w552]
                  disable-tunnel: w540 -> [w549]
                  disable-tunnel: w538 -> [w553]
                  disable-tunnel: w537 -> [w554]
                  disable-tunnel: w532 -> [w562]
                  disable-tunnel: [w558] -> w531
                  disable-tunnel: w529 -> [w559]
                  disable-tunnel: w528 -> [w550]
                  disable-tunnel: w522 -> [w557]
                  frame Enabled {
                    n121 = call "StandAloneTransient_TestBenchParametersArrayCreation.vi"("Input Voltage Array"=w562, "Board Number"=w557, "DUT"=w556, "Nominal Current (A)"=w555, "XINC"=w554, "Test Type"=w553, "Effective LET"=w561, "Sample Rate (SPS)"=w552, "Threshold Percentage (%)"=w551, "Ion (ex. Kr)"=w560, "wfm info single capture"=w550, "Channel"=w559, "Mitigation Information"=w549) -> ("Array"=w558:string[][])  [unwired: 6 in]
                  }
                }
              }
              frame #2 {
                n122 = local read "Channel To Mitigate (0-7) IND"() -> (w572:i32)
                n123 = Add(x=2, y=w572) -> (x+y=w570:i32)
                n124 = local read "number of resets"() -> (w567:i32)
                n125 = Index Array(array=w573, index (row)=w570, index (col)=0 ("disabled index (col)")) -> (element=w569:string)
                n126 = Build Array("Channel_to_mitigate", w569) -> (w575:string[])
                n127 = Number To Decimal String(number=w567) -> (decimal integer string=w566:string)  [unwired: 1 in]
                n128 = Insert Into Array(array=w573, new element=w575) -> (w568:string[][])  [unwired: 2 in]
                n129 = Build Array("Number_of_resets" ("element"), w566) -> (w564:string[])
                n130 = Insert Into Array(array=w568, new element=w564) -> (w563:string[][])  [unwired: 2 in]
              }
              frame #3 {
                n131 = call-poly <vilib>:"Write Delimited Spreadsheet.vi"("file path (dialog if empty)"=w582, "format (%s)"="%s" ("format (%.3f)"), "2D data"=w578, "append to file? (new file:F)"=FALSE, "error in (no error)"=w580, "transpose? (no:F)"=FALSE, "delimiter (\\t)"="," ("delimiter (\\t)")) -> ("error out"=w579:errorcluster)  [unwired: 7 in, 1 out]
              }
              frame #4 {
              }
            }
          }
          frame "HOLDOFF", Default {
            n132 = Equal?(x=w589, y=0) -> (x = y?=w590:bool)
            n133 = local read "INITIALIZED"() -> (w601:bool)
            n134 = Or(x=w590, y="APPLYPATH") -> (x .or. y?=w591:bool)
            n135 = case shown="False" w601 {
              tunnel: w591 -> [w607 _]
              tunnel: w603 -> [w606 w611]
              tunnel: [w605 w611] -> w602
              tunnel: [w604 "FOLDERCREATION"] -> w600
              tunnel: w599 -> [w604 _]
              frame False {
                n136 = case shown="True" w607 {
                  tunnel: w606 -> [w608 _]
                  tunnel: [w608 "INPUTPATH"] -> w605
                  frame False {
                  }
                  frame True {
                  }
                }
              }
              frame True {
              }
            }
          }
        }
        "CURRENTPATH" <- w93
        n137 = local read "FINISH PROGRAM"() -> (w95:bool)
      }
      n138 = while {
        shift-right: [w1869] -> _
        shift-left: "STANDBY" -> [w1871]
        shift-right: [w1867] -> _
        shift-left: FALSE -> [w1868]
        tunnel: "PSU" -> [w1865]
        shift-right: [w1866] -> w48
        shift-left: w25 -> [w1864]
        shift-right: [w1852] -> _
        shift-left: string[][] [["Unconfirmed"]] -> [w1851]
        shift-right: [w1850] -> _
        shift-left: "Unconfirmed" ("read buffer") -> [w1849]
        tunnel: "resource name" -> [w1846]
        shift-right: [w1840] -> _
        shift-left: FALSE -> [w1839]
        i -> [w1836]
        stop <- "stop" stop-if-true
        n139 = Greater?(x=w1836, y=2000000000) -> (0:→"RESTART PROGRAM SOON (DATACOLLECT)":bool)
        n140 = Equal?(x=0, y=w1836) -> (x = y?=w1842:bool)
        n141 = Or(x="APPLY POWER SETTINGS", y=w1842) -> (x .or. y?=w1844:bool)
        n142 = Build Array("Voltage Channel 1", "Voltage Channel 2", "Voltage Channel 3") -> (w1857:dbl[])
        n143 = Build Array("Current Limit Channel 1", "Current Limit Channel 2", "Current Limit Channel 3") -> (w1853:dbl[])
        n144 = case shown="\"POWER_APPLY\"" w1871 {
          tunnel: ["STANDBY" w1918 "STANDBY" "STANDBY" "STANDBY" "STANDBY"] -> w1869
          tunnel: w1868 -> [w1880 w1912 w1998 w2012 w2023 w2032]
          tunnel: [w1879 w1915 w1998 w2012 w2023 w2032] -> w1867
          tunnel: w1864 -> [w1890 w1913 w1995 w2004 w2016 w2025]
          tunnel: [w1889 w1914 w1993 w2003 w2013 w2024] -> w1866
          tunnel: w1865 -> [w1887 _ w1996 _ w2014 _]
          tunnel: "POWER ON" -> [_ w1908 _ _ _ _]
          tunnel: w1844 -> [_ w1911 _ _ _ _]
          tunnel: "Combination" -> [w1878 _ _ _ _ _]
          tunnel: "Channels to Parallelize (if selected)" -> [w1877 _ _ _ _ _]
          tunnel: w1857 -> [w1876 _ _ _ _ _]
          tunnel: w1853 -> [w1875 _ _ _ _ _]
          tunnel: [w1874 w1910 w1991 w2011 w2021 w2031] -> w1852
          tunnel: w1851 -> [_ w1910 w1991 w2011 w2021 w2031]
          tunnel: [w1873 w1909 w1994 w2010 w2020 w2030] -> w1850
          tunnel: w1849 -> [_ w1909 w1994 w2010 w2020 w2030]
          tunnel: w1846 -> [_ _ _ w2007 w2018 w2027]
          tunnel: "NIDCPOWER_CHAN" -> [_ _ _ w2006 w2017 w2026]
          tunnel: "NIDCPOWER_VOLT" -> [_ _ _ w2005 _ _]
          tunnel: "DC Power On" -> [_ w1907 _ _ _ _]
          tunnel: [w1872 w1906 w1992 TRUE FALSE FALSE] -> w1840
          tunnel: w1839 -> [w1872 w1905 w1992 _ _ _]
          frame "POWER_APPLY" {
            # "Creating the Voltage/Current Array that is passed into the keithley 2230 block"
            n145 = Build Array(w1876, w1875) -> (w1892:dbl[][])
            n146 = Transpose 2D Array(2D array=w1892) -> (transposed array=w1891:dbl[][])
            n147 = disable-structure shown="Enabled" {
              disable-tunnel: w1891 -> [w1895]
              disable-tunnel: w1890 -> [w1898]
              disable-tunnel: [w1899] -> w1889
              disable-tunnel: [w1902] -> w1888
              disable-tunnel: w1887 -> [w1894]
              disable-tunnel: [w1901] -> w1886
              disable-tunnel: w1880 -> [w1904]
              disable-tunnel: [w1903] -> w1879
              disable-tunnel: w1878 -> [w1896]
              disable-tunnel: w1877 -> [w1897]
              disable-tunnel: [w1900] -> w1873
              frame Enabled {
                n148 = call "StandAloneTransient_Dynamic_Keithley2230_PSU_Configuration_V1.vi"("VISA resource name"=w1894, "POWER STATUS IN"=w1904, "Input Array (Voltage,Current_Limit)"=w1895, "Combination Scheme"=w1896, "Which Channels to Parallelize"=w1897, "error in"=w1898) -> ("POWER STATUS OUT"=w1903:bool, "Array 4"=w1902:dbl[][], "Array"=w1901:string[], "read buffer"=w1900:string, "error out"=w1899:errorcluster)  [unwired: 5 in]
              }
            }
            n149 = Number To Fractional String(number=w1888) -> (F-format string=w1884:string[][])  [unwired: 3 in]
            n150 = Insert Into Array(array=w1884, index (col)=0 ("disabled index (col)"), new element=w1886) -> (w1881:string[][])  [unwired: 1 in]
            n151 = Insert Into Array(array=w1881, index (row)=0, new element=string[] ["CHANNEL", "VOLTAGE", "CURRENT LIMIT"] ("new element/subarray")) -> (w1874:string[][])  [unwired: 1 in]
          }
          frame "STANDBY", Default {
            n152 = Not(x=w1912) -> (.not. x?=w1916:bool)
            n153 = And(x=w1916, y=w1908) -> (x .and. y?=w1917:bool)
            n154 = case shown="False" w1917 {
              selector: w1917 -> [_ w1990]
              tunnel: [w1933 "POWER_ON"] -> w1918
              tunnel: [w1928 w1990] -> w1915
              tunnel: [w1932 w1988] -> w1914
              tunnel: w1913 -> [w1931 w1988]
              tunnel: w1912 -> [w1930 _]
              tunnel: w1908 -> [w1929 _]
              tunnel: w1911 -> [w1927 _]
              tunnel: w1908 -> [w1926 _]
              tunnel: w1907 -> [w1925 _]
              tunnel: [w1919 w1987] -> w1906
              tunnel: w1905 -> [w1922 w1987]
              tunnel: w1905 -> [w1920 _]
              frame False {
                n155 = And(x=w1925, y=w1926) -> (x .and. y?=w1924:bool)
                n156 = Not(x=w1922) -> (.not. x?=w1921:bool)
                n157 = And(x=w1924, y=w1921) -> (x .and. y?=w1923:bool)
                n158 = case shown="False" w1923 {
                  selector: w1923 -> [w1940 _]
                  tunnel: [w1947 "ENABLE_ON"] -> w1933
                  tunnel: [w1946 w1984] -> w1932
                  tunnel: w1931 -> [w1945 w1984]
                  tunnel: w1930 -> [w1944 w1985]
                  tunnel: w1929 -> [w1943 _]
                  tunnel: [w1942 w1985] -> w1928
                  tunnel: w1927 -> [w1941 _]
                  tunnel: w1925 -> [w1937 _]
                  tunnel: w1922 -> [w1938 _]
                  tunnel: w1920 -> [w1935 w1983]
                  tunnel: [w1939 w1983] -> w1919
                  frame False {
                    n159 = Not And(1:w1937, 2:w1938) -> (0:w1936:bool)
                    n160 = And(x=w1936, y=w1935) -> (x .and. y?=w1934:bool)
                    n161 = case shown="False" w1934 {
                      tunnel: [w1956 "ENABLE_OFF"] -> w1947
                      tunnel: [w1955 w1980] -> w1946
                      tunnel: w1945 -> [w1954 w1980]
                      tunnel: w1944 -> [w1953 w1982]
                      tunnel: w1943 -> [w1952 _]
                      tunnel: [w1951 w1982] -> w1942
                      tunnel: w1941 -> [w1950 _]
                      tunnel: w1940 -> [_ _]
                      tunnel: [w1949 FALSE] -> w1939
                      tunnel: w1935 -> [w1948 _]
                      frame False {
                        n162 = case shown="False" w1950 {
                          tunnel: [w1966 "POWER_APPLY"] -> w1956
                          tunnel: [w1965 w1977] -> w1955
                          tunnel: w1954 -> [w1964 w1977]
                          tunnel: w1953 -> [w1959 w1976]
                          tunnel: w1952 -> [w1961 _]
                          tunnel: [w1960 w1976] -> w1951
                          tunnel: [w1958 w1975] -> w1949
                          tunnel: w1948 -> [w1957 w1975]
                          frame False {
                            n163 = Not(x=w1961) -> (.not. x?=w1963:bool)
                            n164 = And(x=w1963, y=w1959) -> (x .and. y?=w1962:bool)
                            n165 = case shown="True" w1962 {
                              tunnel: ["STANDBY" "POWER_OFF"] -> w1966
                              tunnel: [w1969 w1974] -> w1965
                              tunnel: w1964 -> [w1969 w1974]
                              tunnel: [w1968 FALSE] -> w1960
                              tunnel: w1959 -> [w1968 _]
                              tunnel: [w1967 FALSE] -> w1958
                              tunnel: w1957 -> [w1967 _]
                              frame False {
                              }
                              frame True {
                              }
                            }
                          }
                          frame True {
                          }
                        }
                      }
                      frame True {
                      }
                    }
                  }
                  frame True {
                  }
                }
              }
              frame True {
              }
            }
          }
          frame "POWER_ON" {
            n166 = disable-structure shown="Enabled" {
              disable-tunnel: w1996 -> [w2001]
              disable-tunnel: w1995 -> [w2000]
              disable-tunnel: [w1999] -> w1993
              frame Enabled {
                n167 = call "StandAloneTransient_Keithley2230_PSU_POWER_ON_V1.vi"("error in (no error)"=w2000, "VISA resource name"=w2001) -> ("error out"=w1999:errorcluster)  [unwired: 9 in]
              }
            }
          }
          frame "ENABLE_ON" {
            n168 = call "StandAloneTransient_NIDCPOWER_PSU_POWER_ON_V1.vi"("error in"=w2004, "voltage level"=w2005, "channel name"=w2006, "resource name"=w2007) -> ("error out"=w2003:errorcluster, "current limit"=→"current limit ind":dbl)  [unwired: 6 in]
          }
          frame "POWER_OFF" {
            n169 = call "StandAloneTransient_NIDCPOWER_PSU_POWER_OFF_V1.vi"("error in"=w2016, "channel name"=w2017, "resource name"=w2018) -> ("eRROR OUT"=w2015:errorcluster)  [unwired: 8 in]
            n170 = call "StandAloneTransient_Keithley2230_PSU_POWER_OFF_V1.vi"("error in (no error)"=w2015, "VISA resource name"=w2014) -> ("error out"=w2013:errorcluster)  [unwired: 9 in]
          }
          frame "ENABLE_OFF" {
            n171 = call "StandAloneTransient_NIDCPOWER_PSU_POWER_OFF_V1.vi"("error in"=w2025, "channel name"=w2026, "resource name"=w2027) -> ("eRROR OUT"=w2024:errorcluster)  [unwired: 8 in]
          }
        }
        "POWER STATE" <- w1867
        "Channels Configured and Values" <- w1852
        "Present Channel Configuration" <- w1850
        "ENABLE STATE" <- w1840
        "FINISH PROGRAM" <- "stop"
        "NIDCPOWER_CHAN_CONF" <- "NIDCPOWER_CHAN"
        "NIDCPOWER_VOLT_CONF" <- "NIDCPOWER_VOLT"
      }
      n172 = while {
        shift-right: [w653] -> _
        shift-left: "HOLDBY" -> [w654]
        shift-right: [w651] -> w46
        shift-left: w25 -> [w649]
        tunnel: w50 -> [w650]
        tunnel: [w652] -> w51
        tunnel: w29 -> [w644]
        shift-right: [w628] -> _
        shift-left: 0 ("index") -> [w625]
        shift-right: [w630] -> _
        shift-left: 0.0 ("Nominal Current") -> [w626]
        shift-right: [w629] -> _
        shift-left: 0 ("index") -> [w627]
        shift-right: [w631] -> _
        shift-left: FALSE ("x > y?") -> [w624]
        shift-right: [w623] -> _
        shift-left: 0 -> [w622]
        shift-right: [w621] -> _
        shift-left: T4 {"array"=[], "array"=[], "array"=[], "array"=[], "array"=[], "array"=[], "array"=[], "array"=[]} -> [w620]
        shift-right: [w617] -> _
        shift-left: 3000 ("y") -> [w619]
        shift-right: [w615] -> _
        shift-left: "" -> [w614]
        i -> [w613]
        stop <- w655 stop-if-true
        n173 = Divide(x="TRANSIENT TIME DURATION (ms)", y=1000.0) -> (x/y=w632:dbl)
        n174 = Divide(x="Percent Threshold", y=100.0) -> (x/y=w633:dbl)
        n175 = Greater?(x=w613, y=2000000000) -> (0:→"RESTART PROGRAM SOON (DATASTORE)":bool)
        n176 = case shown="\"COLLECTION16\"" w654 {
          selector: w654 -> [_ _ w973 w1129 _]
          tunnel: [w680 w832 w972 w1131 w1736] -> w653
          tunnel: [w686 w829 w977 w1132 w1735] -> w652
          tunnel: [w685 w828 w974 w1133 w1734] -> w651
          tunnel: w650 -> [w684 w837 w976 w1135 w1735]
          tunnel: w649 -> [w683 w836 w975 w1134 w1734]
          tunnel: "BEGIN RECORDING" -> [_ _ _ w1130 w1733]
          tunnel: "channels" -> [w679 w821 w963 w1128 _]
          tunnel: "Min. Sample Rate" -> [w674 w835 _ _ _]
          tunnel: "Vertical Range (V)" -> [w682 w834 _ _ _]
          tunnel: "Max Points per Fetch" -> [_ _ _ w1127 _]
          tunnel: w644 -> [_ _ _ w1126 _]
          tunnel: "INTIALIZE SCOPE" -> [_ _ _ _ w1732]
          tunnel: "50 ohm vertical range (V)" -> [w678 w830 _ _ _]
          tunnel: "Channel 0 50 ohms?" -> [w677 w831 _ _ _]
          tunnel: "min record length" -> [w675 w827 _ _ _]
          tunnel: "vertical coupling" -> [w676 w826 _ _ _]
          tunnel: w627 -> [_ w823 w967 w1125 w1730]
          tunnel: "Nominal Mitigation Value" -> [_ _ _ w1124 _]
          tunnel: w633 -> [_ _ _ w1123 _]
          tunnel: w632 -> [_ _ _ w1122 _]
          tunnel: w625 -> [_ w822 w968 w1121 w1728]
          tunnel: w626 -> [_ w824 w969 w1120 w1729]
          tunnel: w624 -> [_ w825 w970 w1119 w1731]
          tunnel: [FALSE ("x > y?") w825 w970 w1118 w1731] -> w631
          tunnel: [0.0 ("Nominal Current") w824 w969 w1117 w1729] -> w630
          tunnel: [0 ("index") w823 w967 w1116 w1730] -> w629
          tunnel: [0 ("index") w822 w968 w1115 w1728] -> w628
          tunnel: [w669 w820 w962 w1114 w1727] -> w623
          tunnel: w622 -> [_ _ w962 w1114 w1727]
          tunnel: [T4 {"array"=[], "array"=[], "array"=[], "array"=[], "array"=[], "array"=[], "array"=[], "array"=[]} w819 w966 w1113 w1726] -> w621
          tunnel: w620 -> [_ w819 w966 w1112 w1726]
          tunnel: w613 -> [_ _ _ w1111 _]
          tunnel: w619 -> [_ w818 w965 w1110 w1725]
          tunnel: "Min. Sample Rate" -> [w667 _ _ _ _]
          tunnel: [w664 w818 w965 w1110 w1725] -> w617
          tunnel: [w656 w803 w964 w1109 w1724] -> w615
          tunnel: w614 -> [_ _ w964 w1108 w1724]
          frame "INITIALIZE" {
            n177 = flat-sequence {
              tunnel: w674 -> [w693]
              tunnel: w676 -> [w694]
              tunnel: w677 -> [w695]
              tunnel: w679 -> [w690]
              tunnel: w682 -> [w696]
              tunnel: w683 -> [w688]
              tunnel: w684 -> [w697]
              tunnel: [w697] -> w663
              tunnel: [w687] -> w662
              tunnel: [w696] -> w661
              tunnel: [w689] -> w660
              tunnel: [w695] -> w659
              tunnel: [w694] -> w658
              tunnel: [w693] -> w657
              tunnel: [w782] -> w686
              tunnel: [w781] -> w685
              tunnel: ["WAIT4FOLDER"] -> w681
              tunnel: w678 -> [w764]
              tunnel: w675 -> [w757]
              tunnel: [w755] -> w669
              tunnel: w663 -> [w780]
              tunnel: w662 -> [w779]
              tunnel: w661 -> [w778]
              tunnel: w660 -> [w754]
              tunnel: w659 -> [w763]
              tunnel: w658 -> [w762]
              tunnel: w657 -> [w756]
              tunnel: [w754] -> w656
              frame #0 {
                n178 = while {
                  shift-right: [w713] -> _
                  shift-left: w690 -> [w714]
                  shift-right: [w699] -> _
                  shift-left: 0 -> [w705]
                  shift-right: [w707] -> w689
                  shift-left: "" -> [w703]
                  tunnel: [w713] -> _ mode=indexing
                  tunnel: w688 -> [w702]
                  tunnel: [w701] -> w687
                  i -> [w712]
                  stop <- w711 stop-if-true
                  n179 = flat-sequence {
                    tunnel: w714 -> [w724]
                    tunnel: w712 -> [_]
                    tunnel: [w722] -> w710
                    tunnel: [w715] -> w709
                    tunnel: [w716] -> w708
                    tunnel: [w721] -> w706
                    tunnel: w705 -> [w721]
                    tunnel: [w720] -> w704
                    tunnel: w703 -> [w720]
                    tunnel: [w715] -> w698
                    tunnel: w710 -> [w736]
                    tunnel: w709 -> [w727]
                    tunnel: w708 -> [w735]
                    tunnel: w706 -> [w733]
                    tunnel: w704 -> [w732]
                    tunnel: w702 -> [w731]
                    tunnel: [w736] -> w713
                    tunnel: [w727] -> w711
                    tunnel: [w734] -> w707
                    tunnel: [w730] -> w701
                    tunnel: [w729] -> w700
                    tunnel: w698 -> [w728]
                    frame #0 {
                      n180 = Match Pattern(string=w724, regular expression=",") -> (before substring=w719:string, after substring=w722:string, offset past match=w726:i32)  [unwired: 1 in, 1 out]
                      n181 = Equal?(x=w719, y="") -> (x = y?=w717:bool)
                      n182 = Equal?(x=w726, y=-1) -> (x = y?=w715:bool)
                      n183 = And(x=w715, y=w717) -> (x .and. y?=w716:bool)
                    }
                    frame #1 {
                      n184 = case shown="False" w735 {
                        tunnel: [w737 ""] -> w734
                        tunnel: w733 -> [w742 w751]
                        tunnel: w732 -> [w740 _]
                        tunnel: [w742 w751] -> w729
                        tunnel: w731 -> [w741 _]
                        tunnel: [w741 errorcluster {"status"=TRUE, "code"=-5, "source"="No Channel Parameter: Ensure you have entered channel names in on \"channels (comma separated)\" AND there is no comma at the end of the string in \"channels (comma separated)"} ("error out")] -> w730
                        tunnel: w728 -> [_ _]
                        tunnel: w727 -> [w738 _]
                        frame False {
                          n185 = Number To Decimal String(number=w742) -> (decimal integer string=w739:string)  [unwired: 1 in]
                          n186 = case shown="True" w738 {
                            tunnel: w740 -> [w746 w749]
                            tunnel: w739 -> [w745 w748]
                            tunnel: [w743 w747] -> w737
                            frame False {
                              n187 = Concatenate Strings(w746, w745, "," ("string")) -> (w743:string)
                            }
                            frame True {
                              n188 = Concatenate Strings(w749, w748) -> (w747:string)
                            }
                          }
                        }
                        frame True {
                        }
                      }
                    }
                  }
                  n189 = Increment(x=w700) -> (x+1=w699:i32)
                }
              }
              frame #1 {
                w783 = u32 0 items=["1 mega ohm"=0, "50 ohms"=2] ("input impedance")
                w788 = 388 items=["Start"=482, "Trigger"=483, "Pretrigger"=477, "Now"=481, "Read Pointer"=388] ("Fetch:Fetch Relative To")
                # "3"
                n190 = String Length(string=w754) -> (length=w776:i32)
                n191 = Match Pattern(string=w754, regular expression="0") -> (offset past match=w766:i32)  [unwired: 1 in, 3 out]
                n192 = call <instrlib>:"niScope Configure Vertical.vi"("instrument handle"=w780, "vertical coupling"=w762, "channels"=w754, "vertical range"=w778, "error in"=w779) -> ("instrument handle out"=w785:refnum<k15>, "error out"=w784:errorcluster)  [unwired: 9 in]
                n193 = Quotient & Remainder(x=w776, y=2) -> (x-y*floor(x/y)=w773:i32, floor(x/y)=w774:i32)
                n194 = Not Equal?(x=w766, y=-1) -> (x != y?=w767:bool)
                n195 = And(x=w763, y=w767) -> (x .and. y?=w768:bool)
                n196 = Add(x=w773, y=w774) -> (x+y=w755:i32)
                n197 = call <instrlib>:"niScope Configure Chan Characteristics.vi"("instrument handle"=w785, "channels"=w754, "input impedance"=w783, "maximum input frequency"=0.0, "error in"=w784) -> ("instrument handle out"=w771:refnum<k15>, "error out"=w770:errorcluster)  [unwired: 9 in]
                n198 = case shown="True" w768 {
                  tunnel: [w792 w802] -> w761
                  tunnel: [w791 w801] -> w760
                  tunnel: w771 -> [w792 w796]
                  tunnel: w770 -> [w791 w795]
                  tunnel: w764 -> [_ w793]
                  frame False {
                  }
                  frame True {
                    w799 = u32 2 items=["1 mega ohm"=0, "50 ohms"=2] ("input impedance")
                    w794 = "0" ("channels")
                    n199 = call <instrlib>:"niScope Configure Vertical.vi"("instrument handle"=w796, "channels"=w794, "vertical range"=w793, "error in"=w795) -> ("instrument handle out"=w798:refnum<k15>, "error out"=w797:errorcluster)  [unwired: 10 in]
                    n200 = call <instrlib>:"niScope Configure Chan Characteristics.vi"("instrument handle"=w798, "channels"=w794, "input impedance"=w799, "maximum input frequency"=0.0, "error in"=w797) -> ("instrument handle out"=w802:refnum<k15>, "error out"=w801:errorcluster)  [unwired: 9 in]
                  }
                }
                n201 = call <instrlib>:"niScope Configure Horizontal Timing.vi"("instrument handle"=w761, "min sample rate"=w756, "error in"=w760, "min record length"=w757) -> ("instrument handle out"=w758:refnum<k15>, "error out"=w759:errorcluster)  [unwired: 10 in]
                n202 = call-poly <instrlib>:"niScope Configure Trigger (poly).vi"("instrument handle"=w758, "error in"=w759) -> ("instrument handle out"=w787:refnum<k15>, "error out"=w786:errorcluster)  [unwired: 12 in]
                n203 = call <instrlib>:"niScope Initiate Acquisition.vi"("instrument handle"=w787, "error in"=w786) -> ("instrument handle out"=w789:refnum<k15>, "error out"=w790:errorcluster)  [unwired: 12 in]
                n204 = property class="niScope" props=["Fetch:Fetch Relative To", "Acquisition:Binary Sample Width", "Actual Sample Rate", "Actual Record Length"](reference=w789, error in=w790, "Fetch:Fetch Relative To"=w788) -> (reference out=w782:refnum<k15>, error out=w781:errorcluster, "Actual Sample Rate"=→"Sample Rate IND":dbl)  [unwired: 2 out]
              }
            }
            n205 = Divide(x=15000000.0, y=w667) -> (x/y=w665:dbl)
            n206 = To Long Integer(number=w665) -> (32bit integer=w664:i32)
            n207 = Concatenate Strings(w681) -> (w680:string)
          }
          frame "CONFIGSCOPE" {
            n208 = flat-sequence {
              tunnel: w821 -> [w843]
              tunnel: w826 -> [w844]
              tunnel: w831 -> [w845]
              tunnel: w834 -> [w846]
              tunnel: w835 -> [w847]
              tunnel: w836 -> [w839]
              tunnel: w837 -> [w848]
              tunnel: [w848] -> w817
              tunnel: [w847] -> w815
              tunnel: [w846] -> w813
              tunnel: [w845] -> w811
              tunnel: [w844] -> w809
              tunnel: [w840] -> w807
              tunnel: [w838] -> w804
              tunnel: w817 -> [w910]
              tunnel: [w910] -> w816
              tunnel: w815 -> [w909]
              tunnel: [w909] -> w814
              tunnel: w813 -> [w908]
              tunnel: [w908] -> w812
              tunnel: w811 -> [w907]
              tunnel: [w907] -> w810
              tunnel: w809 -> [w906]
              tunnel: [w906] -> w808
              tunnel: w807 -> [w905]
              tunnel: [w905] -> w806
              tunnel: [w904] -> w805
              tunnel: w804 -> [w904]
              tunnel: ["HOLDBY"] -> w833
              tunnel: w830 -> [w931]
              tunnel: [w927] -> w829
              tunnel: [w926] -> w828
              tunnel: w827 -> [w921]
              tunnel: [w915] -> w820
              tunnel: w816 -> [w946]
              tunnel: w814 -> [w945]
              tunnel: w812 -> [w944]
              tunnel: w810 -> [w932]
              tunnel: w808 -> [w920]
              tunnel: w806 -> [w911]
              tunnel: w805 -> [w912]
              tunnel: [w911] -> w803
              frame #0 {
                n209 = while {
                  shift-right: [w864] -> _
                  shift-left: w843 -> [w865]
                  shift-right: [w850] -> _
                  shift-left: 0 -> [w856]
                  shift-right: [w858] -> w840
                  shift-left: "" -> [w854]
                  tunnel: [w864] -> _ mode=indexing
                  tunnel: w839 -> [w853]
                  tunnel: [w852] -> w838
                  i -> [w863]
                  stop <- w862 stop-if-true
                  n210 = flat-sequence {
                    tunnel: w865 -> [w875]
                    tunnel: w863 -> [_]
                    tunnel: [w873] -> w861
                    tunnel: [w866] -> w860
                    tunnel: [w867] -> w859
                    tunnel: [w872] -> w857
                    tunnel: w856 -> [w872]
                    tunnel: [w871] -> w855
                    tunnel: w854 -> [w871]
                    tunnel: [w866] -> w849
                    tunnel: w861 -> [w887]
                    tunnel: w860 -> [w878]
                    tunnel: w859 -> [w886]
                    tunnel: w857 -> [w884]
                    tunnel: w855 -> [w883]
                    tunnel: w853 -> [w882]
                    tunnel: [w887] -> w864
                    tunnel: [w878] -> w862
                    tunnel: [w885] -> w858
                    tunnel: [w881] -> w852
                    tunnel: [w880] -> w851
                    tunnel: w849 -> [w879]
                    frame #0 {
                      n211 = Match Pattern(string=w875, regular expression=",") -> (before substring=w870:string, after substring=w873:string, offset past match=w877:i32)  [unwired: 1 in, 1 out]
                      n212 = Equal?(x=w870, y="") -> (x = y?=w868:bool)
                      n213 = Equal?(x=w877, y=-1) -> (x = y?=w866:bool)
                      n214 = And(x=w866, y=w868) -> (x .and. y?=w867:bool)
                    }
                    frame #1 {
                      n215 = case shown="False" w886 {
                        tunnel: [w888 ""] -> w885
                        tunnel: w884 -> [w893 w902]
                        tunnel: w883 -> [w891 _]
                        tunnel: [w893 w902] -> w880
                        tunnel: w882 -> [w892 _]
                        tunnel: [w892 errorcluster {"status"=TRUE, "code"=0, "source"="No Channel Parameter"} ("error out")] -> w881
                        tunnel: w879 -> [_ _]
                        tunnel: w878 -> [w889 _]
                        frame False {
                          n216 = Number To Decimal String(number=w893) -> (decimal integer string=w890:string)  [unwired: 1 in]
                          n217 = case shown="False" w889 {
                            tunnel: w891 -> [w897 w900]
                            tunnel: w890 -> [w896 w899]
                            tunnel: [w894 w898] -> w888
                            frame False {
                              n218 = Concatenate Strings(w897, w896, "," ("string")) -> (w894:string)
                            }
                            frame True {
                              n219 = Concatenate Strings(w900, w899) -> (w898:string)
                            }
                          }
                        }
                        frame True {
                        }
                      }
                    }
                  }
                  n220 = Increment(x=w851) -> (x+1=w850:i32)
                }
              }
              frame #1 {
              }
              frame #2 {
                w928 = 388 items=["Start"=482, "Trigger"=483, "Pretrigger"=477, "Now"=481, "Read Pointer"=388] ("Fetch:Fetch Relative To")
                w947 = u32 0 items=["1 mega ohm"=0, "50 ohms"=2] ("input impedance")
                # "3"
                n221 = String Length(string=w911) -> (length=w919:i32)
                n222 = call <instrlib>:"niScope Configure Vertical.vi"("instrument handle"=w946, "vertical coupling"=w920, "channels"=w911, "vertical range"=w944, "error in"=w912) -> ("instrument handle out"=w949:refnum<k15>, "error out"=w948:errorcluster)  [unwired: 9 in]
                n223 = Match Pattern(string=w911, regular expression="0") -> (offset past match=w934:i32)  [unwired: 1 in, 3 out]
                n224 = Quotient & Remainder(x=w919, y=2) -> (x-y*floor(x/y)=w916:i32, floor(x/y)=w917:i32)
                n225 = Not Equal?(x=w934, y=-1) -> (x != y?=w935:bool)
                n226 = And(x=w932, y=w935) -> (x .and. y?=w936:bool)
                n227 = Add(x=w916, y=w917) -> (x+y=w915:i32)
                n228 = call <instrlib>:"niScope Configure Chan Characteristics.vi"("instrument handle"=w949, "channels"=w911, "input impedance"=w947, "maximum input frequency"=0.0, "error in"=w948) -> ("instrument handle out"=w939:refnum<k15>, "error out"=w938:errorcluster)  [unwired: 9 in]
                n229 = case shown="False" w936 {
                  tunnel: [w951 w961] -> w941
                  tunnel: [w950 w960] -> w940
                  tunnel: w939 -> [w951 w955]
                  tunnel: w938 -> [w950 w954]
                  tunnel: w931 -> [_ w952]
                  frame False {
                  }
                  frame True {
                    w958 = u32 2 items=["1 mega ohm"=0, "50 ohms"=2] ("input impedance")
                    w953 = "0" ("channels")
                    n230 = call <instrlib>:"niScope Configure Vertical.vi"("instrument handle"=w955, "channels"=w953, "vertical range"=w952, "error in"=w954) -> ("instrument handle out"=w957:refnum<k15>, "error out"=w956:errorcluster)  [unwired: 10 in]
                    n231 = call <instrlib>:"niScope Configure Chan Characteristics.vi"("instrument handle"=w957, "channels"=w953, "input impedance"=w958, "maximum input frequency"=0.0, "error in"=w956) -> ("instrument handle out"=w961:refnum<k15>, "error out"=w960:errorcluster)  [unwired: 9 in]
                  }
                }
                n232 = call <instrlib>:"niScope Configure Horizontal Timing.vi"("instrument handle"=w941, "min sample rate"=w945, "error in"=w940, "min record length"=w921) -> ("instrument handle out"=w913:refnum<k15>, "error out"=w914:errorcluster)  [unwired: 10 in]
                n233 = call-poly <instrlib>:"niScope Configure Trigger (poly).vi"("instrument handle"=w913, "error in"=w914) -> ("instrument handle out"=w923:refnum<k15>, "error out"=w922:errorcluster)  [unwired: 12 in]
                n234 = call <instrlib>:"niScope Initiate Acquisition.vi"("instrument handle"=w923, "error in"=w922) -> ("instrument handle out"=w929:refnum<k15>, "error out"=w930:errorcluster)  [unwired: 12 in]
                n235 = property class="niScope" props=["Fetch:Fetch Relative To", "Acquisition:Binary Sample Width"](reference=w929, error in=w930, "Fetch:Fetch Relative To"=w928) -> (reference out=w924:refnum<k15>, error out=w925:errorcluster)  [unwired: 1 out]
                n236 = call <instrlib>:"niScope Abort.vi"("instrument handle"=w924, "error in"=w925) -> ("instrument handle out"=w927:refnum<k15>, "error out"=w926:errorcluster)  [unwired: 12 in]
              }
            }
            n237 = Concatenate Strings(w833) -> (w832:string)
          }
          frame "WAIT4FOLDER" {
            n238 = local read "FOLDERCREATED"() -> (w971:bool)
            n239 = case shown="True" w971 {
              tunnel: [w980 w990] -> w977
              tunnel: w976 -> [w980 w992]
              tunnel: w975 -> [w979 w991]
              tunnel: [w979 w989] -> w974
              tunnel: w973 -> [w978 _]
              tunnel: [w978 w988] -> w972
              tunnel: w963 -> [_ w982]
              tunnel: w962 -> [_ w981]
              frame False {
              }
              frame True {
                n240 = flat-sequence {
                  tunnel: w991 -> [w995]
                  tunnel: w992 -> [w996]
                  tunnel: [w996] -> w984
                  tunnel: [w995] -> w983
                  tunnel: w982 -> [w994]
                  tunnel: w981 -> [w993]
                  tunnel: [w1101] -> w987
                  tunnel: [w1100] -> w986
                  tunnel: [w1096] -> w985
                  tunnel: w984 -> [w1103]
                  tunnel: w983 -> [w1102]
                  tunnel: [w1105] -> w988
                  tunnel: [w1106] -> w989
                  tunnel: [w1107] -> w990
                  tunnel: w987 -> [w1107]
                  tunnel: w986 -> [w1106]
                  tunnel: w985 -> [w1105]
                  frame #0 {
                    n241 = case shown="2" w993 {
                      tunnel: w994 -> [_ w998 w1003 w1011 w1021 w1032 w1038 w1054 w1078 _]
                      frame ..0 {
                      }
                      frame 1, Default {
                        w997 = "CHANNEL_NOT_DEFINED" ("CHANNEL 3 NAME")
                        n242 = local write "CHANNEL 0 NAME"(w998) -> ()
                        n243 = local write "CHANNEL 1 NAME"(w997) -> ()
                        n244 = local write "CHANNEL 3 NAME"(w997) -> ()
                        n245 = local write "CHANNEL 4 NAME"(w997) -> ()
                        n246 = local write "CHANNEL 5 NAME"(w997) -> ()
                        n247 = local write "CHANNEL 6 NAME"(w997) -> ()
                        n248 = local write "CHANNEL 7 NAME"(w997) -> ()
                        n249 = local write "CHANNEL 2 NAME"(w997) -> ()
                      }
                      frame 2 {
                        w999 = "CHANNEL_NOT_DEFINED" ("CHANNEL 3 NAME")
                        n250 = Match Pattern(string=w1003, regular expression=",") -> (before substring=w1001:string, after substring=w1000:string)  [unwired: 1 in, 2 out]
                        n251 = local write "CHANNEL 0 NAME"(w1001) -> ()
                        n252 = local write "CHANNEL 1 NAME"(w1000) -> ()
                        n253 = local write "CHANNEL 2 NAME"(w999) -> ()
                        n254 = local write "CHANNEL 4 NAME"(w999) -> ()
                        n255 = local write "CHANNEL 5 NAME"(w999) -> ()
                        n256 = local write "CHANNEL 6 NAME"(w999) -> ()
                        n257 = local write "CHANNEL 7 NAME"(w999) -> ()
                        n258 = local write "CHANNEL 3 NAME"(w999) -> ()
                      }
                      frame 3 {
                        w1004 = "CHANNEL_NOT_DEFINED" ("CHANNEL 3 NAME")
                        n259 = Match Pattern(string=w1011, regular expression=",") -> (before substring=w1009:string, after substring=w1007:string)  [unwired: 1 in, 2 out]
                        n260 = local write "CHANNEL 0 NAME"(w1009) -> ()
                        n261 = Match Pattern(string=w1007, regular expression=",") -> (before substring=w1006:string, after substring=w1005:string)  [unwired: 1 in, 2 out]
                        n262 = local write "CHANNEL 1 NAME"(w1006) -> ()
                        n263 = local write "CHANNEL 2 NAME"(w1005) -> ()
                        n264 = local write "CHANNEL 3 NAME"(w1004) -> ()
                        n265 = local write "CHANNEL 5 NAME"(w1004) -> ()
                        n266 = local write "CHANNEL 6 NAME"(w1004) -> ()
                        n267 = local write "CHANNEL 7 NAME"(w1004) -> ()
                        n268 = local write "CHANNEL 4 NAME"(w1004) -> ()
                      }
                      frame 4 {
                        w1012 = "CHANNEL_NOT_DEFINED" ("CHANNEL 3 NAME")
                        n269 = Match Pattern(string=w1021, regular expression=",") -> (before substring=w1020:string, after substring=w1018:string)  [unwired: 1 in, 2 out]
                        n270 = local write "CHANNEL 0 NAME"(w1020) -> ()
                        n271 = Match Pattern(string=w1018, regular expression=",") -> (before substring=w1017:string, after substring=w1014:string)  [unwired: 1 in, 2 out]
                        n272 = local write "CHANNEL 1 NAME"(w1017) -> ()
                        n273 = Match Pattern(string=w1014, regular expression=",") -> (before substring=w1015:string, after substring=w1013:string)  [unwired: 1 in, 2 out]
                        n274 = local write "CHANNEL 2 NAME"(w1015) -> ()
                        n275 = local write "CHANNEL 3 NAME"(w1013) -> ()
                        n276 = local write "CHANNEL 4 NAME"(w1012) -> ()
                        n277 = local write "CHANNEL 6 NAME"(w1012) -> ()
                        n278 = local write "CHANNEL 7 NAME"(w1012) -> ()
                        n279 = local write "CHANNEL 5 NAME"(w1012) -> ()
                      }
                      frame 5 {
                        w1023 = "CHANNEL_NOT_DEFINED" ("CHANNEL 3 NAME")
                        n280 = Match Pattern(string=w1032, regular expression=",") -> (before substring=w1030:string, after substring=w1031:string)  [unwired: 1 in, 2 out]
                        n281 = local write "CHANNEL 0 NAME"(w1030) -> ()
                        n282 = Match Pattern(string=w1031, regular expression=",") -> (before substring=w1029:string, after substring=w1028:string)  [unwired: 1 in, 2 out]
                        n283 = local write "CHANNEL 1 NAME"(w1029) -> ()
                        n284 = Match Pattern(string=w1028, regular expression=",") -> (before substring=w1027:string, after substring=w1026:string)  [unwired: 1 in, 2 out]
                        n285 = local write "CHANNEL 2 NAME"(w1027) -> ()
                        n286 = Match Pattern(string=w1026, regular expression=",") -> (before substring=w1025:string, after substring=w1024:string)  [unwired: 1 in, 2 out]
                        n287 = local write "CHANNEL 5 NAME"(w1023) -> ()
                        n288 = local write "CHANNEL 7 NAME"(w1023) -> ()
                        n289 = local write "CHANNEL 6 NAME"(w1023) -> ()
                        n290 = local write "CHANNEL 3 NAME"(w1025) -> ()
                        n291 = local write "CHANNEL 4 NAME"(w1024) -> ()
                      }
                      frame 6 {
                        w1037 = "CHANNEL_NOT_DEFINED" ("CHANNEL 3 NAME")
                        n292 = Match Pattern(string=w1038, regular expression=",") -> (before substring=w1048:string, after substring=w1047:string)  [unwired: 1 in, 2 out]
                        n293 = local write "CHANNEL 0 NAME"(w1048) -> ()
                        n294 = Match Pattern(string=w1047, regular expression=",") -> (before substring=w1046:string, after substring=w1044:string)  [unwired: 1 in, 2 out]
                        n295 = local write "CHANNEL 1 NAME"(w1046) -> ()
                        n296 = Match Pattern(string=w1044, regular expression=",") -> (before substring=w1045:string, after substring=w1043:string)  [unwired: 1 in, 2 out]
                        n297 = local write "CHANNEL 2 NAME"(w1045) -> ()
                        n298 = Match Pattern(string=w1043, regular expression=",") -> (before substring=w1042:string, after substring=w1041:string)  [unwired: 1 in, 2 out]
                        n299 = local write "CHANNEL 6 NAME"(w1037) -> ()
                        n300 = local write "CHANNEL 7 NAME"(w1037) -> ()
                        n301 = local write "CHANNEL 3 NAME"(w1042) -> ()
                        n302 = Match Pattern(string=w1041, regular expression=",") -> (before substring=w1039:string, after substring=w1040:string)  [unwired: 1 in, 2 out]
                        n303 = local write "CHANNEL 4 NAME"(w1039) -> ()
                        n304 = local write "CHANNEL 5 NAME"(w1040) -> ()
                      }
                      frame 8 {
                        n305 = Match Pattern(string=w1054, regular expression=",") -> (before substring=w1068:string, after substring=w1067:string)  [unwired: 1 in, 2 out]
                        n306 = local write "CHANNEL 0 NAME"(w1068) -> ()
                        n307 = Match Pattern(string=w1067, regular expression=",") -> (before substring=w1066:string, after substring=w1065:string)  [unwired: 1 in, 2 out]
                        n308 = local write "CHANNEL 1 NAME"(w1066) -> ()
                        n309 = Match Pattern(string=w1065, regular expression=",") -> (before substring=w1064:string, after substring=w1063:string)  [unwired: 1 in, 2 out]
                        n310 = local write "CHANNEL 2 NAME"(w1064) -> ()
                        n311 = Match Pattern(string=w1063, regular expression=",") -> (before substring=w1062:string, after substring=w1061:string)  [unwired: 1 in, 2 out]
                        n312 = local write "CHANNEL 3 NAME"(w1062) -> ()
                        n313 = Match Pattern(string=w1061, regular expression=",") -> (before substring=w1060:string, after substring=w1059:string)  [unwired: 1 in, 2 out]
                        n314 = local write "CHANNEL 4 NAME"(w1060) -> ()
                        n315 = Match Pattern(string=w1059, regular expression=",") -> (before substring=w1058:string, after substring=w1057:string)  [unwired: 1 in, 2 out]
                        n316 = local write "CHANNEL 5 NAME"(w1058) -> ()
                        n317 = Match Pattern(string=w1057, regular expression=",") -> (before substring=w1056:string, after substring=w1055:string)  [unwired: 1 in, 2 out]
                        n318 = local write "CHANNEL 6 NAME"(w1056) -> ()
                        n319 = local write "CHANNEL 7 NAME"(w1055) -> ()
                      }
                      frame 7 {
                        n320 = Match Pattern(string=w1078, regular expression=",") -> (before substring=w1089:string, after substring=w1088:string)  [unwired: 1 in, 2 out]
                        n321 = local write "CHANNEL 0 NAME"(w1089) -> ()
                        n322 = Match Pattern(string=w1088, regular expression=",") -> (before substring=w1087:string, after substring=w1086:string)  [unwired: 1 in, 2 out]
                        n323 = local write "CHANNEL 1 NAME"(w1087) -> ()
                        n324 = Match Pattern(string=w1086, regular expression=",") -> (before substring=w1085:string, after substring=w1084:string)  [unwired: 1 in, 2 out]
                        n325 = local write "CHANNEL 2 NAME"(w1085) -> ()
                        n326 = Match Pattern(string=w1084, regular expression=",") -> (before substring=w1083:string, after substring=w1082:string)  [unwired: 1 in, 2 out]
                        n327 = local write "CHANNEL 7 NAME"("CHANNEL_NOT_DEFINED" ("CHANNEL 3 NAME")) -> ()
                        n328 = local write "CHANNEL 3 NAME"(w1083) -> ()
                        n329 = Match Pattern(string=w1082, regular expression=",") -> (before substring=w1081:string, after substring=w1080:string)  [unwired: 1 in, 2 out]
                        n330 = local write "CHANNEL 4 NAME"(w1081) -> ()
                        n331 = Match Pattern(string=w1080, regular expression=",") -> (before substring=w1079:string, after substring=w1077:string)  [unwired: 1 in, 2 out]
                        n332 = local write "CHANNEL 5 NAME"(w1079) -> ()
                        n333 = local write "CHANNEL 6 NAME"(w1077) -> ()
                      }
                      frame 9.. {
                      }
                    }
                  }
                  frame #1 {
                    n334 = property class="niScope"(reference=w1103, error in=w1102) -> (reference out=w1101:refnum<k15>, error out=w1100:errorcluster, "Acquisition:Binary Sample Width"=w1098:i32)
                    n335 = Number To Decimal String(number=w1098) -> (decimal integer string=w1097:string)  [unwired: 1 in]
                    n336 = Concatenate Strings("COLLECTION", w1097) -> (w1096:string)
                  }
                  frame #2 {
                    n337 = local write "FOLDERCREATED"(FALSE) -> ()
                  }
                }
              }
            }
          }
          frame "COLLECTION16" {
            n338 = case shown="True" w1130 {
              tunnel: w1135 -> [w1145 w1236]
              tunnel: w1134 -> [w1144 w1235]
              tunnel: [w1142 w1233] -> w1133
              tunnel: [w1143 w1228] -> w1132
              tunnel: ["HOLDOFF" w1149] -> w1131
              tunnel: w1129 -> [_ w1149]
              tunnel: w1128 -> [_ _]
              tunnel: w1127 -> [_ w1234]
              tunnel: w1126 -> [_ w1182]
              tunnel: w1125 -> [w1140 w1227]
              tunnel: w1124 -> [_ w1224]
              tunnel: w1123 -> [_ w1222]
              tunnel: w1122 -> [_ w1220]
              tunnel: w1121 -> [w1138 w1218]
              tunnel: w1120 -> [w1139 w1216]
              tunnel: w1119 -> [w1141 w1214]
              tunnel: [w1141 w1213] -> w1118
              tunnel: [w1139 w1212] -> w1117
              tunnel: [w1140 w1211] -> w1116
              tunnel: [w1138 w1210] -> w1115
              tunnel: w1114 -> [_ w1208]
              tunnel: [w1137 w1207] -> w1113
              tunnel: w1112 -> [w1137 w1205]
              tunnel: w1111 -> [_ w1150]
              tunnel: w1110 -> [_ w1151]
              tunnel: [w1136 w1148] -> w1109
              tunnel: w1108 -> [w1136 w1148]
              frame False {
                n339 = call <instrlib>:"niScope Abort.vi"("instrument handle"=w1145, "error in"=w1144) -> ("instrument handle out"=w1143:refnum<k15>, "error out"=w1142:errorcluster)  [unwired: 12 in]
              }
              frame True {
                n340 = flat-sequence {
                  tunnel: w1234 -> [w1255]
                  tunnel: [w1237] -> _
                  tunnel: w1235 -> [w1256]
                  tunnel: w1236 -> [w1257]
                  tunnel: [w1257] -> w1232
                  tunnel: [w1256] -> w1231
                  tunnel: [w1237] -> w1230
                  tunnel: [w1255] -> w1229
                  tunnel: w1227 -> [w1253]
                  tunnel: [w1253] -> w1226
                  tunnel: [w1252] -> w1225
                  tunnel: w1224 -> [w1252]
                  tunnel: [w1251] -> w1223
                  tunnel: w1222 -> [w1251]
                  tunnel: [w1250] -> w1221
                  tunnel: w1220 -> [w1250]
                  tunnel: [w1249] -> w1219
                  tunnel: w1218 -> [w1249]
                  tunnel: [w1248] -> w1217
                  tunnel: w1216 -> [w1248]
                  tunnel: [w1247] -> w1215
                  tunnel: w1214 -> [w1247]
                  tunnel: [w1246] -> w1209
                  tunnel: w1208 -> [w1246]
                  tunnel: w1205 -> [w1245]
                  tunnel: [w1245] -> w1206
                  tunnel: w1150 -> [w1240]
                  tunnel: [w1239] -> w1152
                  tunnel: w1151 -> [w1238]
                  tunnel: w1148 -> [w1237]
                  tunnel: w1232 -> [w1275]
                  tunnel: w1231 -> [w1274]
                  tunnel: w1230 -> [w1273]
                  tunnel: w1229 -> [w1272]
                  tunnel: [w1261] -> w1181
                  tunnel: [w1271] -> w1179
                  tunnel: [w1259] -> w1177
                  tunnel: [w1260] -> w1175
                  tunnel: w1226 -> [w1270]
                  tunnel: [w1270] -> w1173
                  tunnel: [w1269] -> w1171
                  tunnel: w1225 -> [w1269]
                  tunnel: [w1268] -> w1169
                  tunnel: w1223 -> [w1268]
                  tunnel: [w1267] -> w1167
                  tunnel: w1221 -> [w1267]
                  tunnel: w1219 -> [w1266]
                  tunnel: [w1266] -> w1165
                  tunnel: [w1265] -> w1163
                  tunnel: w1217 -> [w1265]
                  tunnel: [w1264] -> w1161
                  tunnel: w1215 -> [w1264]
                  tunnel: w1209 -> [w1263]
                  tunnel: [w1263] -> w1159
                  tunnel: w1206 -> [w1262]
                  tunnel: [w1262] -> w1157
                  tunnel: [w1259] -> w1155
                  tunnel: [w1258] -> w1153
                  tunnel: w1152 -> [w1258]
                  tunnel: w1181 -> [w1294]
                  tunnel: [w1294] -> w1180
                  tunnel: w1179 -> [w1293]
                  tunnel: [w1293] -> w1178
                  tunnel: w1177 -> [w1292]
                  tunnel: [w1292] -> w1176
                  tunnel: w1175 -> [w1291]
                  tunnel: [w1291] -> w1174
                  tunnel: w1173 -> [w1290]
                  tunnel: [w1290] -> w1172
                  tunnel: w1171 -> [w1289]
                  tunnel: [w1289] -> w1170
                  tunnel: w1169 -> [w1288]
                  tunnel: [w1288] -> w1168
                  tunnel: w1167 -> [w1287]
                  tunnel: [w1287] -> w1166
                  tunnel: w1165 -> [w1286]
                  tunnel: [w1286] -> w1164
                  tunnel: w1163 -> [w1285]
                  tunnel: [w1285] -> w1162
                  tunnel: w1161 -> [w1284]
                  tunnel: [w1284] -> w1160
                  tunnel: w1159 -> [w1283]
                  tunnel: [w1283] -> w1158
                  tunnel: w1157 -> [w1280]
                  tunnel: [w1281] -> w1156
                  tunnel: w1155 -> [w1282]
                  tunnel: [w1282] -> w1154
                  tunnel: w1153 -> [w1279]
                  tunnel: [w1277] -> w1147
                  tunnel: w1180 -> [w1347]
                  tunnel: w1178 -> [w1346]
                  tunnel: w1176 -> [w1315]
                  tunnel: w1174 -> [w1311]
                  tunnel: w1172 -> [w1326]
                  tunnel: w1170 -> [w1324]
                  tunnel: w1168 -> [w1323]
                  tunnel: w1166 -> [w1325]
                  tunnel: w1164 -> [w1322]
                  tunnel: w1162 -> [w1320]
                  tunnel: w1160 -> [w1321]
                  tunnel: [w1347] -> w1204
                  tunnel: [w1346] -> w1202
                  tunnel: [w1319] -> w1200
                  tunnel: [w1318] -> w1198
                  tunnel: [w1317] -> w1196
                  tunnel: [w1316] -> w1194
                  tunnel: [w1311] -> w1192
                  tunnel: [w1315] -> w1190
                  tunnel: [w1314] -> w1188
                  tunnel: w1158 -> [w1314]
                  tunnel: [w1313] -> w1186
                  tunnel: w1156 -> [w1313]
                  tunnel: [w1312] -> w1184
                  tunnel: w1154 -> [w1312]
                  tunnel: [w1311] -> w1183
                  tunnel: w1147 -> [w1307]
                  tunnel: w1204 -> [w1424]
                  tunnel: [w1423] -> w1203
                  tunnel: w1202 -> [w1432]
                  tunnel: [w1432] -> w1201
                  tunnel: w1200 -> [w1431]
                  tunnel: [w1431] -> w1199
                  tunnel: w1198 -> [w1430]
                  tunnel: [w1430] -> w1197
                  tunnel: w1196 -> [w1419]
                  tunnel: [w1419] -> w1195
                  tunnel: w1194 -> [w1429]
                  tunnel: [w1429] -> w1193
                  tunnel: w1192 -> [w1428]
                  tunnel: [w1428] -> w1191
                  tunnel: w1190 -> [w1427]
                  tunnel: [w1427] -> w1189
                  tunnel: w1188 -> [w1426]
                  tunnel: [w1426] -> w1187
                  tunnel: w1186 -> [w1425]
                  tunnel: [w1425] -> w1185
                  tunnel: w1184 -> [w1422]
                  tunnel: w1183 -> [w1421]
                  tunnel: w1182 -> [w1416]
                  tunnel: [w1441] -> w1210
                  tunnel: [w1442] -> w1211
                  tunnel: [w1443] -> w1212
                  tunnel: [w1444] -> w1213
                  tunnel: [w1445] -> w1228
                  tunnel: [w1436] -> w1233
                  tunnel: w1203 -> [w1440]
                  tunnel: w1201 -> [w1445]
                  tunnel: w1199 -> [w1444]
                  tunnel: w1197 -> [w1443]
                  tunnel: w1195 -> [w1442]
                  tunnel: w1193 -> [w1441]
                  tunnel: w1191 -> [w1439]
                  tunnel: w1189 -> [w1438]
                  tunnel: w1187 -> [w1437]
                  tunnel: [w1435] -> w1207
                  tunnel: w1185 -> [w1434]
                  frame #0 {
                    n341 = Quotient & Remainder(x=w1240, y=w1238) -> (x-y*floor(x/y)=w1243:i32, floor(x/y)=w1244:i32)
                    n342 = Equal To 0?(x=w1243) -> (x = 0?=w1242:bool)
                    n343 = Not Equal To 0?(x=w1244) -> (x != 0?=w1241:bool)
                    n344 = And(x=w1242, y=w1241) -> (x .and. y?=w1239:bool)
                    n345 = Wait (ms)(milliseconds to wait="milliseconds to wait") -> ()  [unwired: 1 out]
                  }
                  frame #1 {
                    w1276 = 0.0  # timeout
                    n346 = call-poly <instrlib>:"niScope Fetch (poly).vi"("timeout"=w1276, "error in"=w1274, "numSamples"=w1272, "channels"=w1273, "instrument handle"=w1275) -> ("error out"=w1261:errorcluster, "wfm"=w1260:i16[][], "wfm info"=w1259:T2, "instrument handle out"=w1271:refnum<k15>)  [unwired: 3 in]
                    "wfm info IND" <- w1259
                  }
                  frame #2 {
                    n347 = case shown="True" w1279 {
                      tunnel: [w1295 w1296] -> w1281
                      tunnel: w1280 -> [w1295 _]
                      frame False {
                      }
                      frame True {
                        n348 = Bundle("array"=dbl[] [], "array"=dbl[] [], "array"=dbl[] [], "array"=dbl[] [], "array"=dbl[] [], "array"=dbl[] [], "array"=dbl[] [], "array"=dbl[] []) -> (w1296:T4)  [unwired: 1 in]
                      }
                    }
                    n349 = local read "IndicatorOutputs"() -> (w1278:cluster{"Run Information":string, string})
                    n350 = Unbundle(w1278) -> (w1277:string)  [unwired: 1 out]
                  }
                  frame #3 {
                    # "shift register"
                    # "SHIFT REGISTER"
                    n351 = Increment(x=w1323) -> (x+1=w1336:dbl)
                    n352 = Negate(x=w1323) -> (-x=w1335:dbl)
                    n353 = Index Array(array=w1311, index (row)=0 ("index")) -> (element=w1329:i16[])  [unwired: 1 in]
                    n354 = Multiply(x=w1324, y=w1336) -> (x*y=w1306:dbl)
                    n355 = Increment(x=w1335) -> (x+1=w1334:dbl)
                    n356 = Array Size(array=w1329) -> (size(s)=w1328:i32)
                    "Last Point Fetched" <- w1328
                    n357 = Add(x=w1328, y=w1326) -> (x+y=→"Total Points Fetched":i32)
                    n358 = Multiply(x=w1324, y=w1334) -> (x*y=w1309:dbl)
                    n359 = Index Array(array=w1315, index="Channel To Mitigate (0-7)") -> (element=w1345:T9)
                    n360 = Index Array(array=w1311, index (row)="Channel To Mitigate (0-7)") -> (element=w1342:i16[])  [unwired: 1 in]
                    n361 = Unbundle By Name(w1345) -> ("actualSamples"=→"NUMBER SAMPLES":i32, "xIncrement"=→"XINC":dbl, "absoluteInitialX"=w1344:dbl)
                    n362 = Unbundle By Name(w1345) -> ("gain"=w1340:dbl, "offset"=w1338:dbl)
                    n363 = To Double Precision Float(number=w1342) -> (double precision float=w1341:dbl[])
                    n364 = Multiply(x=w1340, y=w1341) -> (x*y=w1339:dbl[])
                    n365 = Add(x=w1338, y=w1339) -> (x+y=w1337:dbl[])
                    n366 = case shown="\"Latchup\", Default" w1307 {
                      tunnel: w1337 -> [w1349 w1357]
                      tunnel: [w1350 w1355] -> w1310
                      tunnel: w1309 -> [_ w1353]
                      tunnel: [w1351 w1354] -> w1308
                      tunnel: w1306 -> [w1348 _]
                      tunnel: [w1348 w1353] -> w1305
                      frame "Latchup", Default {
                        n367 = Array Max & Min(array=w1349) -> (max value=w1352:dbl, max index (indices)=w1350:i32)  [unwired: 2 out]
                        n368 = Greater?(x=w1352, y=w1348) -> (0:w1351:bool)
                      }
                      frame "Transient" {
                        # "shift register"
                        n369 = Array Max & Min(array=w1357) -> (min value=w1356:dbl, min index (indices)=w1355:i32)  [unwired: 2 out]
                        n370 = Greater?(x=w1353, y=w1356) -> (0:w1354:bool)
                      }
                    }
                    "EXCEED THRESHOLD" <- w1308
                    "Threshold Value" <- w1305
                    n371 = disable-structure shown="Enabled" {
                      disable-tunnel: w1308 -> [w1369 w1415]
                      disable-tunnel: w1344 -> [w1368 _]
                      disable-tunnel: [w1367 w1415] -> w1343
                      disable-tunnel: w1325 -> [w1366 _]
                      disable-tunnel: w1322 -> [w1365 w1414]
                      disable-tunnel: w1321 -> [w1364 _]
                      disable-tunnel: w1320 -> [w1363 _]
                      disable-tunnel: [w1362 _] -> w1319
                      disable-tunnel: [w1361 _] -> w1318
                      disable-tunnel: [w1360 w1413] -> w1317
                      disable-tunnel: [w1359 w1414] -> w1316
                      disable-tunnel: w1310 -> [w1358 w1413]
                      frame Enabled {
                        n372 = case shown="True" w1369 {
                          selector: w1369 -> [w1373 w1387]
                          tunnel: w1365 -> [w1370 w1378]
                          tunnel: w1358 -> [_ w1376]
                          tunnel: [-1 w1375] -> w1360
                          tunnel: w1368 -> [_ w1383]
                          tunnel: w1364 -> [_ w1385]
                          tunnel: [w1373 w1387] -> w1362
                          tunnel: [0.0 w1382] -> w1361
                          tunnel: w1363 -> [_ w1381]
                          tunnel: w1366 -> [_ w1380]
                          tunnel: [FALSE w1379] -> w1367
                          tunnel: [w1370 w1377] -> w1359
                          frame False {
                          }
                          frame True {
                            n373 = Not(x=w1385) -> (.not. x?=w1386:bool)
                            n374 = And(x=w1386, y=w1387) -> (x .and. y?=w1384:bool)
                            n375 = case shown="False" w1384 {
                              tunnel: w1383 -> [w1398 w1412]
                              tunnel: [w1394 w1411] -> w1382
                              tunnel: w1381 -> [w1388 _]
                              tunnel: w1380 -> [w1396 _]
                              tunnel: [w1393 FALSE] -> w1379
                              tunnel: w1378 -> [w1392 w1409]
                              tunnel: [w1391 w1409] -> w1377
                              tunnel: [w1390 -1] -> w1375
                              tunnel: w1376 -> [w1389 _]
                              frame False {
                                n376 = Add(x=w1388, y=w1398) -> (x+y=w1395:dbl)
                                n377 = Greater?(x=w1395, y=w1396) -> (0:w1397:bool)
                                n378 = case shown="True" w1397 {
                                selector: w1397 -> [w1402 w1406]
                                tunnel: w1395 -> [_ _]
                                tunnel: [w1399 0.0] -> w1394
                                tunnel: [w1402 w1406] -> w1393
                                tunnel: w1392 -> [w1401 w1405]
                                tunnel: [w1401 w1404] -> w1391
                                tunnel: [-1 w1403] -> w1390
                                tunnel: w1389 -> [_ w1403]
                                tunnel: w1388 -> [w1399 _]
                                frame False {
                                }
                                frame True {
                                n379 = Increment(x=w1405) -> (x+1=w1404:i32)
                                }
                                }
                              }
                              frame True {
                                n380 = Negate(x=w1412) -> (-x=w1411:dbl)
                              }
                            }
                          }
                        }
                      }
                      frame Disabled {
                      }
                    }
                    "Over Threshold Number" <- w1316
                    "EXCEED DURATION" <- w1343
                    "Percent Threshold IND" <- w1323
                    "Nominal Current IND" <- w1324
                    "Channel To Mitigate (0-7) IND" <- "Channel To Mitigate (0-7)"
                  }
                  frame #4 {
                    (unwired) T8 {"wfm info"=[], "wfm"=[]} ("cluster")
                    n381 = Bundle(cluster=T5 {"wfm info"=[], "wfm"=[], "Beam On?"=FALSE, 0}, "wfm info"=w1422, "wfm"=w1421, "Beam On?"="Beam On?", w1419) -> (w1417:T5)
                    n382 = Enqueue Element(queue=w1416, element=w1417, error in (no error)=w1424) -> (error out=w1423:errorcluster)  [unwired: 1 in, 2 out]
                  }
                  frame #5 {
                    n383 = case shown="True" "Plot Data?" {
                      tunnel: w1437 -> [_ w1454]
                      tunnel: w1438 -> [_ w1453]
                      tunnel: w1439 -> [_ w1452]
                      tunnel: [w1447 w1451] -> w1436
                      tunnel: w1440 -> [w1447 w1450]
                      tunnel: [w1446 w1449] -> w1435
                      tunnel: w1434 -> [w1446 w1448]
                      frame False {
                      }
                      frame True {
                        n384 = case shown="8" w1454 {
                          tunnel: w1453 -> [_ w1471 w1493 w1518 w1546 w1580 w1616 w1658 w1703 _]
                          tunnel: w1452 -> [_ w1470 w1492 w1517 w1547 w1579 w1617 w1657 w1702 _]
                          tunnel: [w1456 w1469 w1491 w1516 w1545 w1578 w1615 w1656 w1701 w1723] -> w1451
                          tunnel: w1450 -> [w1456 w1469 w1491 w1516 w1545 w1578 w1615 w1656 w1701 w1723]
                          tunnel: [w1455 w1457 w1477 w1500 w1527 w1558 w1593 w1647 w1686 w1722] -> w1449
                          tunnel: w1448 -> [w1455 w1466 w1486 w1509 w1536 w1569 w1602 w1640 w1683 w1722]
                          frame ..0 {
                          }
                          frame 1, Default {
                            n385 = disable-structure shown="Enabled" {
                              disable-tunnel: 0 ("index") -> [w1474]
                              disable-tunnel: w1471 -> [w1475]
                              disable-tunnel: w1470 -> [w1473]
                              disable-tunnel: [w1476] -> w1468
                              frame Enabled {
                                n386 = call "StandAloneTransient_SingleGraphCreation_DataCollection_Light.vi"("wfm"=w1473, "index"=w1474, "wfm info"=w1475) -> ("Array"=w1476:dbl[])  [unwired: 8 in]
                              }
                            }
                            n387 = Unbundle(w1466) -> ("array"=w1465:dbl[], "array"=w1464:dbl[], "array"=w1463:dbl[], "array"=w1462:dbl[], "array"=w1461:dbl[], "array"=w1460:dbl[], "array"=w1459:dbl[], "array"=w1458:dbl[])
                            n388 = local write "Channel Graph 0"(w1468) -> ()
                            n389 = Insert Into Array(array=w1465, new element=w1468) -> (w1467:dbl[])  [unwired: 1 in]
                            n390 = local write "Channel Graph Cumulative 0"(w1467) -> ()
                            n391 = Bundle("array"=w1467, "array"=w1464, "array"=w1463, "array"=w1462, "array"=w1461, "array"=w1460, "array"=w1459, "array"=w1458) -> (w1457:T4)  [unwired: 1 in]
                          }
                          frame 2 {
                            n392 = disable-structure shown="Enabled" {
                              disable-tunnel: w1493 -> [w1496]
                              disable-tunnel: w1492 -> [w1497]
                              disable-tunnel: [w1495] -> w1490
                              disable-tunnel: [w1494] -> w1489
                              frame Enabled {
                                n393 = call "StandAloneTransient_SingleGraphCreation_DataCollection_Light.vi"("wfm"=w1497, "index"=0, "wfm info"=w1496) -> ("Array"=w1495:dbl[])  [unwired: 8 in]
                                n394 = call "StandAloneTransient_SingleGraphCreation_DataCollection_Light.vi"("wfm"=w1497, "index"=1, "wfm info"=w1496) -> ("Array"=w1494:dbl[])  [unwired: 8 in]
                              }
                            }
                            n395 = Unbundle(w1486) -> ("array"=w1485:dbl[], "array"=w1484:dbl[], "array"=w1483:dbl[], "array"=w1482:dbl[], "array"=w1481:dbl[], "array"=w1480:dbl[], "array"=w1479:dbl[], "array"=w1478:dbl[])
                            n396 = local write "Channel Graph 1"(w1489) -> ()
                            n397 = local write "Channel Graph 0"(w1490) -> ()
                            n398 = Insert Into Array(array=w1485, new element=w1489) -> (w1488:dbl[])  [unwired: 1 in]
                            n399 = Insert Into Array(array=w1484, new element=w1489) -> (w1487:dbl[])  [unwired: 1 in]
                            n400 = local write "Channel Graph Cumulative 0"(w1488) -> ()
                            n401 = local write "Channel Graph Cumulative 1"(w1487) -> ()
                            n402 = Bundle("array"=w1488, "array"=w1487, "array"=w1483, "array"=w1482, "array"=w1481, "array"=w1480, "array"=w1479, "array"=w1478) -> (w1477:T4)  [unwired: 1 in]
                          }
                          frame 3 {
                            n403 = disable-structure shown="Enabled" {
                              disable-tunnel: w1518 -> [w1523]
                              disable-tunnel: w1517 -> [w1522]
                              disable-tunnel: [w1526] -> w1515
                              disable-tunnel: [w1525] -> w1514
                              disable-tunnel: [w1524] -> w1513
                              frame Enabled {
                                n404 = call "StandAloneTransient_SingleGraphCreation_DataCollection_Light.vi"("wfm"=w1522, "index"=1, "wfm info"=w1523) -> ("Array"=w1525:dbl[])  [unwired: 8 in]
                                n405 = call "StandAloneTransient_SingleGraphCreation_DataCollection_Light.vi"("wfm"=w1522, "index"=2, "wfm info"=w1523) -> ("Array"=w1524:dbl[])  [unwired: 8 in]
                                n406 = call "StandAloneTransient_SingleGraphCreation_DataCollection_Light.vi"("wfm"=w1522, "index"=0, "wfm info"=w1523) -> ("Array"=w1526:dbl[])  [unwired: 8 in]
                              }
                            }
                            n407 = Unbundle(w1509) -> ("array"=w1508:dbl[], "array"=w1507:dbl[], "array"=w1506:dbl[], "array"=w1505:dbl[], "array"=w1504:dbl[], "array"=w1503:dbl[], "array"=w1502:dbl[], "array"=w1501:dbl[])
                            n408 = local write "Channel Graph 2"(w1513) -> ()
                            n409 = local write "Channel Graph 1"(w1514) -> ()
                            n410 = local write "Channel Graph 0"(w1515) -> ()
                            n411 = Insert Into Array(array=w1507, new element=w1514) -> (w1511:dbl[])  [unwired: 1 in]
                            n412 = Insert Into Array(array=w1506, new element=w1513) -> (w1510:dbl[])  [unwired: 1 in]
                            n413 = Insert Into Array(array=w1508, new element=w1515) -> (w1512:dbl[])  [unwired: 1 in]
                            n414 = local write "Channel Graph Cumulative 1"(w1511) -> ()
                            n415 = local write "Channel Graph Cumulative 2"(w1510) -> ()
                            n416 = local write "Channel Graph Cumulative 0"(w1512) -> ()
                            n417 = Bundle("array"=w1512, "array"=w1511, "array"=w1510, "array"=w1505, "array"=w1504, "array"=w1503, "array"=w1502, "array"=w1501) -> (w1500:T4)  [unwired: 1 in]
                          }
                          frame 4 {
                            n418 = disable-structure shown="Enabled" {
                              disable-tunnel: w1547 -> [w1557]
                              disable-tunnel: w1546 -> [w1556]
                              disable-tunnel: [w1548] -> w1544
                              disable-tunnel: [w1549] -> w1543
                              disable-tunnel: [w1550] -> w1542
                              disable-tunnel: [w1551] -> w1541
                              frame Enabled {
                                n419 = call "StandAloneTransient_SingleGraphCreation_DataCollection_Light.vi"("wfm"=w1557, "index"=2, "wfm info"=w1556) -> ("Array"=w1550:dbl[])  [unwired: 8 in]
                                n420 = call "StandAloneTransient_SingleGraphCreation_DataCollection_Light.vi"("wfm"=w1557, "index"=1, "wfm info"=w1556) -> ("Array"=w1549:dbl[])  [unwired: 8 in]
                                n421 = call "StandAloneTransient_SingleGraphCreation_DataCollection_Light.vi"("wfm"=w1557, "index"=3, "wfm info"=w1556) -> ("Array"=w1551:dbl[])  [unwired: 8 in]
                                n422 = call "StandAloneTransient_SingleGraphCreation_DataCollection_Light.vi"("wfm"=w1557, "index"=0, "wfm info"=w1556) -> ("Array"=w1548:dbl[])  [unwired: 8 in]
                              }
                            }
                            "Channel 0 Reference Values" <- w1544
                            n423 = Unbundle(w1536) -> ("array"=w1535:dbl[], "array"=w1534:dbl[], "array"=w1533:dbl[], "array"=w1532:dbl[], "array"=w1531:dbl[], "array"=w1530:dbl[], "array"=w1529:dbl[], "array"=w1528:dbl[])
                            n424 = local write "Channel Graph 2"(w1542) -> ()
                            n425 = local write "Channel Graph 3"(w1541) -> ()
                            n426 = local write "Channel Graph 0"(w1544) -> ()
                            n427 = local write "Channel Graph 1"(w1543) -> ()
                            n428 = Insert Into Array(array=w1534, new element=w1543) -> (w1539:dbl[])  [unwired: 1 in]
                            n429 = Insert Into Array(array=w1533, new element=w1542) -> (w1538:dbl[])  [unwired: 1 in]
                            n430 = Insert Into Array(array=w1535, new element=w1544) -> (w1540:dbl[])  [unwired: 1 in]
                            n431 = Insert Into Array(array=w1532, new element=w1541) -> (w1537:dbl[])  [unwired: 1 in]
                            n432 = local write "Channel Graph Cumulative 1"(w1539) -> ()
                            n433 = local write "Channel Graph Cumulative 2"(w1538) -> ()
                            n434 = local write "Channel Graph Cumulative 0"(w1540) -> ()
                            n435 = local write "Channel Graph Cumulative 3"(w1537) -> ()
                            n436 = Bundle("array"=w1540, "array"=w1539, "array"=w1538, "array"=w1537, "array"=w1531, "array"=w1530, "array"=w1529, "array"=w1528) -> (w1527:T4)  [unwired: 1 in]
                          }
                          frame 5 {
                            n437 = disable-structure shown="Enabled" {
                              disable-tunnel: w1580 -> [w1586]
                              disable-tunnel: w1579 -> [w1592]
                              disable-tunnel: [w1587] -> w1577
                              disable-tunnel: [w1588] -> w1576
                              disable-tunnel: [w1589] -> w1575
                              disable-tunnel: [w1590] -> w1574
                              disable-tunnel: [w1591] -> w1573
                              frame Enabled {
                                n438 = call "StandAloneTransient_SingleGraphCreation_DataCollection_Light.vi"("wfm"=w1592, "index"=2, "wfm info"=w1586) -> ("Array"=w1589:dbl[])  [unwired: 8 in]
                                n439 = call "StandAloneTransient_SingleGraphCreation_DataCollection_Light.vi"("wfm"=w1592, "index"=3, "wfm info"=w1586) -> ("Array"=w1590:dbl[])  [unwired: 8 in]
                                n440 = call "StandAloneTransient_SingleGraphCreation_DataCollection_Light.vi"("wfm"=w1592, "index"=0, "wfm info"=w1586) -> ("Array"=w1587:dbl[])  [unwired: 8 in]
                                n441 = call "StandAloneTransient_SingleGraphCreation_DataCollection_Light.vi"("wfm"=w1592, "index"=1, "wfm info"=w1586) -> ("Array"=w1588:dbl[])  [unwired: 8 in]
                                n442 = call "StandAloneTransient_SingleGraphCreation_DataCollection_Light.vi"("wfm"=w1592, "index"=4, "wfm info"=w1586) -> ("Array"=w1591:dbl[])  [unwired: 8 in]
                              }
                            }
                            n443 = Unbundle(w1569) -> ("array"=w1568:dbl[], "array"=w1567:dbl[], "array"=w1566:dbl[], "array"=w1565:dbl[], "array"=w1564:dbl[], "array"=w1561:dbl[], "array"=w1560:dbl[], "array"=w1559:dbl[])
                            n444 = local write "Channel Graph 1"(w1576) -> ()
                            n445 = local write "Channel Graph 3"(w1574) -> ()
                            n446 = local write "Channel Graph 4"(w1573) -> ()
                            n447 = local write "Channel Graph 0"(w1577) -> ()
                            n448 = local write "Channel Graph 2"(w1575) -> ()
                            n449 = Insert Into Array(array=w1566, new element=w1575) -> (w1570:dbl[])  [unwired: 1 in]
                            n450 = Insert Into Array(array=w1565, new element=w1574) -> (w1563:dbl[])  [unwired: 1 in]
                            n451 = Insert Into Array(array=w1568, new element=w1577) -> (w1572:dbl[])  [unwired: 1 in]
                            n452 = Insert Into Array(array=w1567, new element=w1576) -> (w1571:dbl[])  [unwired: 1 in]
                            n453 = Insert Into Array(array=w1564, new element=w1573) -> (w1562:dbl[])  [unwired: 1 in]
                            n454 = local write "Channel Graph Cumulative 2"(w1570) -> ()
                            n455 = local write "Channel Graph Cumulative 3"(w1563) -> ()
                            n456 = local write "Channel Graph Cumulative 0"(w1572) -> ()
                            n457 = local write "Channel Graph Cumulative 1"(w1571) -> ()
                            n458 = local write "Channel Graph Cumulative 4"(w1562) -> ()
                            n459 = Bundle("array"=w1572, "array"=w1571, "array"=w1570, "array"=w1563, "array"=w1562, "array"=w1561, "array"=w1560, "array"=w1559) -> (w1558:T4)  [unwired: 1 in]
                          }
                          frame 6 {
                            n460 = disable-structure shown="Enabled" {
                              disable-tunnel: w1617 -> [w1631]
                              disable-tunnel: w1616 -> [w1629]
                              disable-tunnel: [w1623] -> w1614
                              disable-tunnel: [w1622] -> w1613
                              disable-tunnel: [w1621] -> w1612
                              disable-tunnel: [w1620] -> w1611
                              disable-tunnel: [w1619] -> w1610
                              disable-tunnel: [w1618] -> w1609
                              frame Enabled {
                                n461 = call "StandAloneTransient_SingleGraphCreation_DataCollection_Light.vi"("wfm"=w1631, "index"=2, "wfm info"=w1629) -> ("Array"=w1621:dbl[])  [unwired: 8 in]
                                n462 = call "StandAloneTransient_SingleGraphCreation_DataCollection_Light.vi"("wfm"=w1631, "index"=3, "wfm info"=w1629) -> ("Array"=w1620:dbl[])  [unwired: 8 in]
                                n463 = call "StandAloneTransient_SingleGraphCreation_DataCollection_Light.vi"("wfm"=w1631, "index"=0, "wfm info"=w1629) -> ("Array"=w1623:dbl[])  [unwired: 8 in]
                                n464 = call "StandAloneTransient_SingleGraphCreation_DataCollection_Light.vi"("wfm"=w1631, "index"=1, "wfm info"=w1629) -> ("Array"=w1622:dbl[])  [unwired: 8 in]
                                n465 = call "StandAloneTransient_SingleGraphCreation_DataCollection_Light.vi"("wfm"=w1631, "index"=4, "wfm info"=w1629) -> ("Array"=w1619:dbl[])  [unwired: 8 in]
                                n466 = call "StandAloneTransient_SingleGraphCreation_DataCollection_Light.vi"("wfm"=w1631, "index"=5, "wfm info"=w1629) -> ("Array"=w1618:dbl[])  [unwired: 8 in]
                              }
                            }
                            n467 = Unbundle(w1602) -> ("array"=w1601:dbl[], "array"=w1600:dbl[], "array"=w1599:dbl[], "array"=w1598:dbl[], "array"=w1597:dbl[], "array"=w1596:dbl[], "array"=w1594:dbl[], "array"=w1595:dbl[])
                            n468 = local write "Channel Graph 1"(w1613) -> ()
                            n469 = local write "Channel Graph 4"(w1610) -> ()
                            n470 = local write "Channel Graph 3"(w1611) -> ()
                            n471 = local write "Channel Graph 5"(w1609) -> ()
                            n472 = local write "Channel Graph 0"(w1614) -> ()
                            n473 = local write "Channel Graph 2"(w1612) -> ()
                            n474 = Insert Into Array(array=w1599, new element=w1612) -> (w1606:dbl[])  [unwired: 1 in]
                            n475 = Insert Into Array(array=w1598, new element=w1611) -> (w1605:dbl[])  [unwired: 1 in]
                            n476 = Insert Into Array(array=w1601, new element=w1614) -> (w1608:dbl[])  [unwired: 1 in]
                            n477 = Insert Into Array(array=w1600, new element=w1613) -> (w1607:dbl[])  [unwired: 1 in]
                            n478 = Insert Into Array(array=w1597, new element=w1610) -> (w1604:dbl[])  [unwired: 1 in]
                            n479 = Insert Into Array(array=w1596, new element=w1609) -> (w1603:dbl[])  [unwired: 1 in]
                            n480 = local write "Channel Graph Cumulative 2"(w1606) -> ()
                            n481 = local write "Channel Graph Cumulative 3"(w1605) -> ()
                            n482 = local write "Channel Graph Cumulative 0"(w1608) -> ()
                            n483 = local write "Channel Graph Cumulative 1"(w1607) -> ()
                            n484 = local write "Channel Graph Cumulative 4"(w1604) -> ()
                            n485 = local write "Channel Graph Cumulative 5"(w1603) -> ()
                            n486 = Bundle("array"=w1608, "array"=w1607, "array"=w1606, "array"=w1605, "array"=w1604, "array"=w1603, "array"=w1594, "array"=w1595) -> (w1593:T4)  [unwired: 1 in]
                          }
                          frame 7 {
                            n487 = disable-structure shown="Enabled" {
                              disable-tunnel: w1658 -> [w1673]
                              disable-tunnel: w1657 -> [w1672]
                              disable-tunnel: [w1674] -> w1655
                              disable-tunnel: [w1671] -> w1654
                              disable-tunnel: [w1670] -> w1653
                              disable-tunnel: [w1669] -> w1652
                              disable-tunnel: [w1668] -> w1651
                              disable-tunnel: [w1667] -> w1650
                              disable-tunnel: [w1666] -> w1649
                              frame Enabled {
                                n488 = call "StandAloneTransient_SingleGraphCreation_DataCollection_Light.vi"("wfm"=w1672, "index"=3, "wfm info"=w1673) -> ("Array"=w1669:dbl[])  [unwired: 8 in]
                                n489 = call "StandAloneTransient_SingleGraphCreation_DataCollection_Light.vi"("wfm"=w1672, "index"=4, "wfm info"=w1673) -> ("Array"=w1668:dbl[])  [unwired: 8 in]
                                n490 = call "StandAloneTransient_SingleGraphCreation_DataCollection_Light.vi"("wfm"=w1672, "index"=0, "wfm info"=w1673) -> ("Array"=w1674:dbl[])  [unwired: 8 in]
                                n491 = call "StandAloneTransient_SingleGraphCreation_DataCollection_Light.vi"("wfm"=w1672, "index"=1, "wfm info"=w1673) -> ("Array"=w1671:dbl[])  [unwired: 8 in]
                                n492 = call "StandAloneTransient_SingleGraphCreation_DataCollection_Light.vi"("wfm"=w1672, "index"=2, "wfm info"=w1673) -> ("Array"=w1670:dbl[])  [unwired: 8 in]
                                n493 = call "StandAloneTransient_SingleGraphCreation_DataCollection_Light.vi"("wfm"=w1672, "index"=5, "wfm info"=w1673) -> ("Array"=w1667:dbl[])  [unwired: 8 in]
                                n494 = call "StandAloneTransient_SingleGraphCreation_DataCollection_Light.vi"("wfm"=w1672, "index"=6, "wfm info"=w1673) -> ("Array"=w1666:dbl[])  [unwired: 8 in]
                              }
                            }
                            n495 = Unbundle(w1640) -> ("array"=w1639:dbl[], "array"=w1638:dbl[], "array"=w1637:dbl[], "array"=w1636:dbl[], "array"=w1635:dbl[], "array"=w1634:dbl[], "array"=w1633:dbl[], "array"=w1632:dbl[])
                            n496 = local write "Channel Graph 2"(w1653) -> ()
                            n497 = local write "Channel Graph 1"(w1654) -> ()
                            n498 = local write "Channel Graph 5"(w1650) -> ()
                            n499 = local write "Channel Graph 6"(w1649) -> ()
                            n500 = local write "Channel Graph 0"(w1655) -> ()
                            n501 = local write "Channel Graph 3"(w1652) -> ()
                            n502 = local write "Channel Graph 4"(w1651) -> ()
                            n503 = Insert Into Array(array=w1636, new element=w1652) -> (w1644:dbl[])  [unwired: 1 in]
                            n504 = Insert Into Array(array=w1635, new element=w1651) -> (w1643:dbl[])  [unwired: 1 in]
                            n505 = Insert Into Array(array=w1639, new element=w1655) -> (w1648:dbl[])  [unwired: 1 in]
                            n506 = Insert Into Array(array=w1638, new element=w1654) -> (w1646:dbl[])  [unwired: 1 in]
                            n507 = Insert Into Array(array=w1637, new element=w1653) -> (w1645:dbl[])  [unwired: 1 in]
                            n508 = Insert Into Array(array=w1634, new element=w1650) -> (w1642:dbl[])  [unwired: 1 in]
                            n509 = Insert Into Array(array=w1633, new element=w1649) -> (w1641:dbl[])  [unwired: 1 in]
                            n510 = local write "Channel Graph Cumulative 3"(w1644) -> ()
                            n511 = local write "Channel Graph Cumulative 4"(w1643) -> ()
                            n512 = local write "Channel Graph Cumulative 0"(w1648) -> ()
                            n513 = local write "Channel Graph Cumulative 1"(w1646) -> ()
                            n514 = local write "Channel Graph Cumulative 2"(w1645) -> ()
                            n515 = local write "Channel Graph Cumulative 5"(w1642) -> ()
                            n516 = local write "Channel Graph Cumulative 6"(w1641) -> ()
                            n517 = Bundle("array"=w1648, "array"=w1646, "array"=w1645, "array"=w1644, "array"=w1643, "array"=w1642, "array"=w1641, "array"=w1632) -> (w1647:T4)  [unwired: 1 in]
                          }
                          frame 8 {
                            n518 = disable-structure shown="Enabled" {
                              disable-tunnel: w1703 -> [w1720]
                              disable-tunnel: w1702 -> [w1721]
                              disable-tunnel: [w1704] -> w1700
                              disable-tunnel: [w1705] -> w1699
                              disable-tunnel: [w1706] -> w1698
                              disable-tunnel: [w1707] -> w1697
                              disable-tunnel: [w1708] -> w1696
                              disable-tunnel: [w1709] -> w1695
                              disable-tunnel: [w1710] -> w1694
                              disable-tunnel: [w1711] -> w1693
                              frame Enabled {
                                n519 = call "StandAloneTransient_SingleGraphCreation_DataCollection_Light.vi"("wfm"=w1721, "index"=3, "wfm info"=w1720) -> ("Array"=w1707:dbl[])  [unwired: 8 in]
                                n520 = call "StandAloneTransient_SingleGraphCreation_DataCollection_Light.vi"("wfm"=w1721, "index"=4, "wfm info"=w1720) -> ("Array"=w1708:dbl[])  [unwired: 8 in]
                                n521 = call "StandAloneTransient_SingleGraphCreation_DataCollection_Light.vi"("wfm"=w1721, "index"=0, "wfm info"=w1720) -> ("Array"=w1704:dbl[])  [unwired: 8 in]
                                n522 = call "StandAloneTransient_SingleGraphCreation_DataCollection_Light.vi"("wfm"=w1721, "index"=1, "wfm info"=w1720) -> ("Array"=w1705:dbl[])  [unwired: 8 in]
                                n523 = call "StandAloneTransient_SingleGraphCreation_DataCollection_Light.vi"("wfm"=w1721, "index"=2, "wfm info"=w1720) -> ("Array"=w1706:dbl[])  [unwired: 8 in]
                                n524 = call "StandAloneTransient_SingleGraphCreation_DataCollection_Light.vi"("wfm"=w1721, "index"=5, "wfm info"=w1720) -> ("Array"=w1709:dbl[])  [unwired: 8 in]
                                n525 = call "StandAloneTransient_SingleGraphCreation_DataCollection_Light.vi"("wfm"=w1721, "index"=6, "wfm info"=w1720) -> ("Array"=w1710:dbl[])  [unwired: 8 in]
                                n526 = call "StandAloneTransient_SingleGraphCreation_DataCollection_Light.vi"("wfm"=w1721, "index"=7, "wfm info"=w1720) -> ("Array"=w1711:dbl[])  [unwired: 8 in]
                              }
                            }
                            n527 = Unbundle(w1683) -> ("array"=w1682:dbl[], "array"=w1681:dbl[], "array"=w1680:dbl[], "array"=w1679:dbl[], "array"=w1678:dbl[], "array"=w1677:dbl[], "array"=w1676:dbl[], "array"=w1675:dbl[])
                            n528 = local write "Channel Graph 2"(w1698) -> ()
                            n529 = local write "Channel Graph 5"(w1695) -> ()
                            n530 = local write "Channel Graph 1"(w1699) -> ()
                            n531 = local write "Channel Graph 6"(w1694) -> ()
                            n532 = local write "Channel Graph 7"(w1693) -> ()
                            n533 = local write "Channel Graph 0"(w1700) -> ()
                            n534 = local write "Channel Graph 3"(w1697) -> ()
                            n535 = local write "Channel Graph 4"(w1696) -> ()
                            n536 = Insert Into Array(array=w1679, new element=w1697) -> (w1689:dbl[])  [unwired: 1 in]
                            n537 = Insert Into Array(array=w1678, new element=w1696) -> (w1688:dbl[])  [unwired: 1 in]
                            n538 = Insert Into Array(array=w1682, new element=w1700) -> (w1692:dbl[])  [unwired: 1 in]
                            n539 = Insert Into Array(array=w1681, new element=w1699) -> (w1691:dbl[])  [unwired: 1 in]
                            n540 = Insert Into Array(array=w1680, new element=w1698) -> (w1690:dbl[])  [unwired: 1 in]
                            n541 = Insert Into Array(array=w1677, new element=w1695) -> (w1687:dbl[])  [unwired: 1 in]
                            n542 = Insert Into Array(array=w1676, new element=w1694) -> (w1685:dbl[])  [unwired: 1 in]
                            n543 = Insert Into Array(array=w1675, new element=w1693) -> (w1684:dbl[])  [unwired: 1 in]
                            n544 = local write "Channel Graph Cumulative 3"(w1689) -> ()
                            n545 = local write "Channel Graph Cumulative 4"(w1688) -> ()
                            n546 = local write "Channel Graph Cumulative 0"(w1692) -> ()
                            n547 = local write "Channel Graph Cumulative 1"(w1691) -> ()
                            n548 = local write "Channel Graph Cumulative 2"(w1690) -> ()
                            n549 = local write "Channel Graph Cumulative 5"(w1687) -> ()
                            n550 = local write "Channel Graph Cumulative 6"(w1685) -> ()
                            n551 = local write "Channel Graph Cumulative 7"(w1684) -> ()
                            n552 = Bundle("array"=w1692, "array"=w1691, "array"=w1690, "array"=w1689, "array"=w1688, "array"=w1687, "array"=w1685, "array"=w1684) -> (w1686:T4)  [unwired: 1 in]
                          }
                          frame 9.. {
                          }
                        }
                      }
                    }
                  }
                }
              }
            }
            "Collecting Data" <- w1130
          }
          frame "HOLDBY", Default {
            n553 = case shown="False" w1733 {
              tunnel: [w1738 "INITIALIZE"] -> w1736
              tunnel: w1732 -> [w1737 _]
              frame False {
                n554 = case shown="False" w1737 {
                  tunnel: ["HOLDBY" "CONFIGSCOPE"] -> w1738
                  frame False {
                  }
                  frame True {
                  }
                }
              }
              frame True {
              }
            }
            "RECORDING DATA" <- w1733
            "INITIALIZED" <- w1733
          }
        }
        "Number Of Channels" <- w623
        "Num Loop 4 Reset Graph" <- w617
        n555 = local read "FINISH PROGRAM"() -> (w655:bool)
        "Min. Sample Rate IND" <- "Min. Sample Rate"
        "channels IND" <- "channels"
        "Vertical Range (V) IND" <- "Vertical Range (V)"
      }
      n556 = while {
        tunnel: "PSU" -> [w1758]
        shift-right: [w1760] -> w21
        shift-left: w25 -> [w1759]
        tunnel: [w1758] -> _
        shift-right: [w1756] -> _
        shift-left: "NONE" -> [w1757]
        tunnel: "resource name" -> [w1755]
        shift-right: [w1742] -> _
        shift-left: 0 -> [w1746]
        stop <- w1761 stop-if-true
        # "ADD THE AUTOMITIGATION PARAMETERS WITHIN THE TEST BENCH"
        n557 = local read "FOLDERCREATED"() -> (w1743:bool)
        n558 = case shown="True" w1743 {
          tunnel: [w1762 0] -> w1745
          tunnel: w1746 -> [w1762 _]
          frame False {
          }
          frame True {
          }
        }
        n559 = local read "EXCEED DURATION"() -> (w1749:bool)
        n560 = local read "Collecting Data"() -> (w1744:bool)
        n561 = And(x="AUTOMITIGATION ENABLED", y=w1744) -> (x .and. y?=w1747:bool)
        n562 = And(x=w1747, y=w1749) -> (x .and. y?=w1750:bool)
        n563 = Or(x="FORCED RESET", y=w1750) -> (x .or. y?=w1751:bool)
        n564 = case shown="False" "CHANGE MITIGATION" {
          tunnel: w1751 -> [w1772 _]
          tunnel: [w1766 w1830] -> w1760
          tunnel: w1759 -> [w1771 w1830]
          tunnel: w1757 -> [w1770 _]
          tunnel: w1758 -> [w1769 _]
          tunnel: [w1768 w1831] -> w1756
          tunnel: w1755 -> [w1767 _]
          tunnel: "Mitigation" -> [_ w1829]
          tunnel: w1745 -> [w1765 w1828]
          tunnel: [w1764 w1828] -> w1742
          frame False {
            n565 = case shown="True" w1772 {
              tunnel: w1769 -> [_ w1785]
              tunnel: [w1775 w1784] -> w1766
              tunnel: w1771 -> [w1775 w1783]
              tunnel: w1770 -> [w1774 w1782]
              tunnel: [w1774 w1781] -> w1768
              tunnel: w1767 -> [_ w1780]
              tunnel: [w1773 w1776] -> w1764
              tunnel: w1765 -> [w1773 w1777]
              frame False {
              }
              frame True {
                n566 = local read "NIDCPOWER_CHAN_CONF"() -> (w1779:string)
                n567 = local read "NIDCPOWER_VOLT_CONF"() -> (w1778:dbl)
                n568 = case shown="\"Hardware\"" w1782 {
                  selector: w1782 -> [w1797 w1809 w1812 w1821]
                  tunnel: w1785 -> [w1794 w1806 _ _]
                  tunnel: [w1786 w1798 w1811 w1818] -> w1784
                  tunnel: w1783 -> [w1792 w1804 w1811 w1819]
                  tunnel: [w1797 w1809 w1812 w1821] -> w1781
                  tunnel: w1780 -> [w1790 w1802 _ w1820]
                  tunnel: w1779 -> [w1789 w1801 _ w1816]
                  tunnel: w1778 -> [w1788 w1800 _ w1815]
                  tunnel: [w1795 w1807 w1810 w1813] -> w1776
                  tunnel: w1777 -> [w1796 w1808 w1810 w1814]
                  frame "PowerCycle" {
                    n569 = call "StandAloneTransient_NIDCPOWER_PSU_POWER_OFF_V1.vi"("error in"=w1792, "channel name"=w1789, "resource name"=w1790) -> ("eRROR OUT"=w1791:errorcluster)  [unwired: 8 in]
                    n570 = Increment(x=w1796) -> (x+1=w1795:i32)
                    n571 = call "StandAloneTransient_Keithley2230_PSU_POWER_CYCLE_V1.vi"("error in (no error)"=w1791, "milliseconds to wait"=u32 200, "VISA Refnum in"=w1794) -> ("error out"=w1787:errorcluster)  [unwired: 8 in]
                    n572 = call "StandAloneTransient_NIDCPOWER_PSU_POWER_ON_V1.vi"("error in"=w1787, "voltage level"=w1788, "channel name"=w1789, "resource name"=w1790) -> ("error out"=w1786:errorcluster)  [unwired: 6 in, 1 out]
                  }
                  frame "Hardware" {
                    n573 = call "StandAloneTransient_NIDCPOWER_PSU_POWER_OFF_V1.vi"("error in"=w1804, "channel name"=w1801, "resource name"=w1802) -> ("eRROR OUT"=w1803:errorcluster)  [unwired: 8 in]
                    n574 = Increment(x=w1808) -> (x+1=w1807:i32)
                    n575 = call "StandAloneTransient_Keithley2230_PSU_POWER_CYCLE_V1.vi"("error in (no error)"=w1803, "milliseconds to wait"=u32 200, "VISA Refnum in"=w1806) -> ("error out"=w1799:errorcluster)  [unwired: 8 in]
                    n576 = call "StandAloneTransient_NIDCPOWER_PSU_POWER_ON_V1.vi"("error in"=w1799, "voltage level"=w1800, "channel name"=w1801, "resource name"=w1802) -> ("error out"=w1798:errorcluster)  [unwired: 6 in, 1 out]
                  }
                  frame "NONE", Default {
                  }
                  frame "EnableCircuit" {
                    n577 = disable-structure shown="Enabled" {
                      disable-tunnel: w1820 -> [w1826]
                      disable-tunnel: w1819 -> [w1823]
                      disable-tunnel: [w1822] -> w1818
                      disable-tunnel: u32 200 ("milliseconds to wait") -> [w1824]
                      disable-tunnel: w1816 -> [w1825]
                      disable-tunnel: w1815 -> [w1827]
                      frame Enabled {
                        n578 = call "StandAloneTransient_NIDCPOWER_PSU_POWER_CYCLE_V1.vi"("NIDCPOWER_VOLT_CONF"=w1827, "error in (no error)"=w1823, "milliseconds to wait"=w1824, "NIDCPOWER_CHAN_CONF"=w1825, "IVI Refnum in"=w1826) -> ("error out"=w1822:errorcluster)  [unwired: 6 in]
                      }
                    }
                    n579 = Increment(x=w1814) -> (x+1=w1813:i32)
                  }
                }
              }
            }
          }
          frame True {
            n580 = case shown="3" w1829 {
              tunnel: ["NONE" "HARDWARE" "EnableCircuit" "PowerCycle"] -> w1831
              frame 0, Default {
              }
              frame 1 {
              }
              frame 3 {
              }
              frame 2 {
              }
            }
          }
        }
        "Present Mitigation Information" <- w1756
        "number of resets" <- w1742
        n581 = local read "FINISH PROGRAM"() -> (w1761:bool)
        "AUTOMITIGATION ENABLED IND" <- "AUTOMITIGATION ENABLED"
      }
      n582 = Release Queue(queue=w29, error in (no error)=w46) -> (error out=w45:errorcluster)  [unwired: 1 in, 2 out]
      n583 = call <instrlib>:"niScope Close.vi"("instrument handle"=w51, "error in"=w45) -> ("error out"=w47:errorcluster)  [unwired: 13 in]
      n584 = VISA Close(VISA resource name=w17, error in (no error)=w19) -> (error out=w18:errorcluster)
      n585 = Merge Errors(w18, w21) -> (w20:errorcluster)
      n586 = Merge Errors(w48, w47, w20) -> (w16:errorcluster)
    }
  }
  n587 = call <vilib>:"Simple Error Handler.vi"("error in (no error)"=w1) -> ()  [unwired: 4 in, 5 out]
